vi "Main_ConfigDialog.vi"(8 "error in (no error)":errorcluster, 9 "boot path":path, 10 "Current project Path":path) -> (0 "error out":errorcluster)   [LabVIEW 2011]
uses:
  signal type.ctl
  gain.ctl
  filter.ctl
  Power_config.ctl
  contable.ctl
  CHS.ctl
  singlechtype.ctl
  <vilib>/Utility/miscctls.llb/LVPositionTypeDef.ctl
  config table enum.ctl
  config opr.ctl
panel:
  out "Numeric":i32
  out "size(s)":i32
  in  "LED":bool
  in  "threshold":dbl
  in  "CALclass":T1
  in  "PHName":string(combo)
  in  "ClassII":string
  in  "ClassI":string
  in  "boardName":string
  in  "Ch":u8
  in  "CNO":u8
  in  "Cluster":T2 {"CHS"."display" format="%b"}
  in  "Load":bool
  in  "Power":T5
  in  "Filter":T6={"en"=FALSE, "value"=10, "Boolean"=FALSE} caption="滤波"
  in  "Gain":T7
  in  "compare":T1
  in  "Apply":bool
  in  "sensorName":string(combo)
  in  "rate":dbl
  in  "alarm":string(combo)
  in  "enable":string(combo)
  in  "b":dbl
  in  "k":dbl
  in  "unit":string(combo)="A"
  in  "Etype":string(combo)="温度"
  in  "ChannalName":string
  in  "ChannalConfig":string(tree)
  in  "OK":bool
  in  "Save as":bool
  in  "Cancel":bool
  # "通道参数配置表"
  # "Ssdsa"
  # "Hz"
  # "Hz"
  # "Hz"
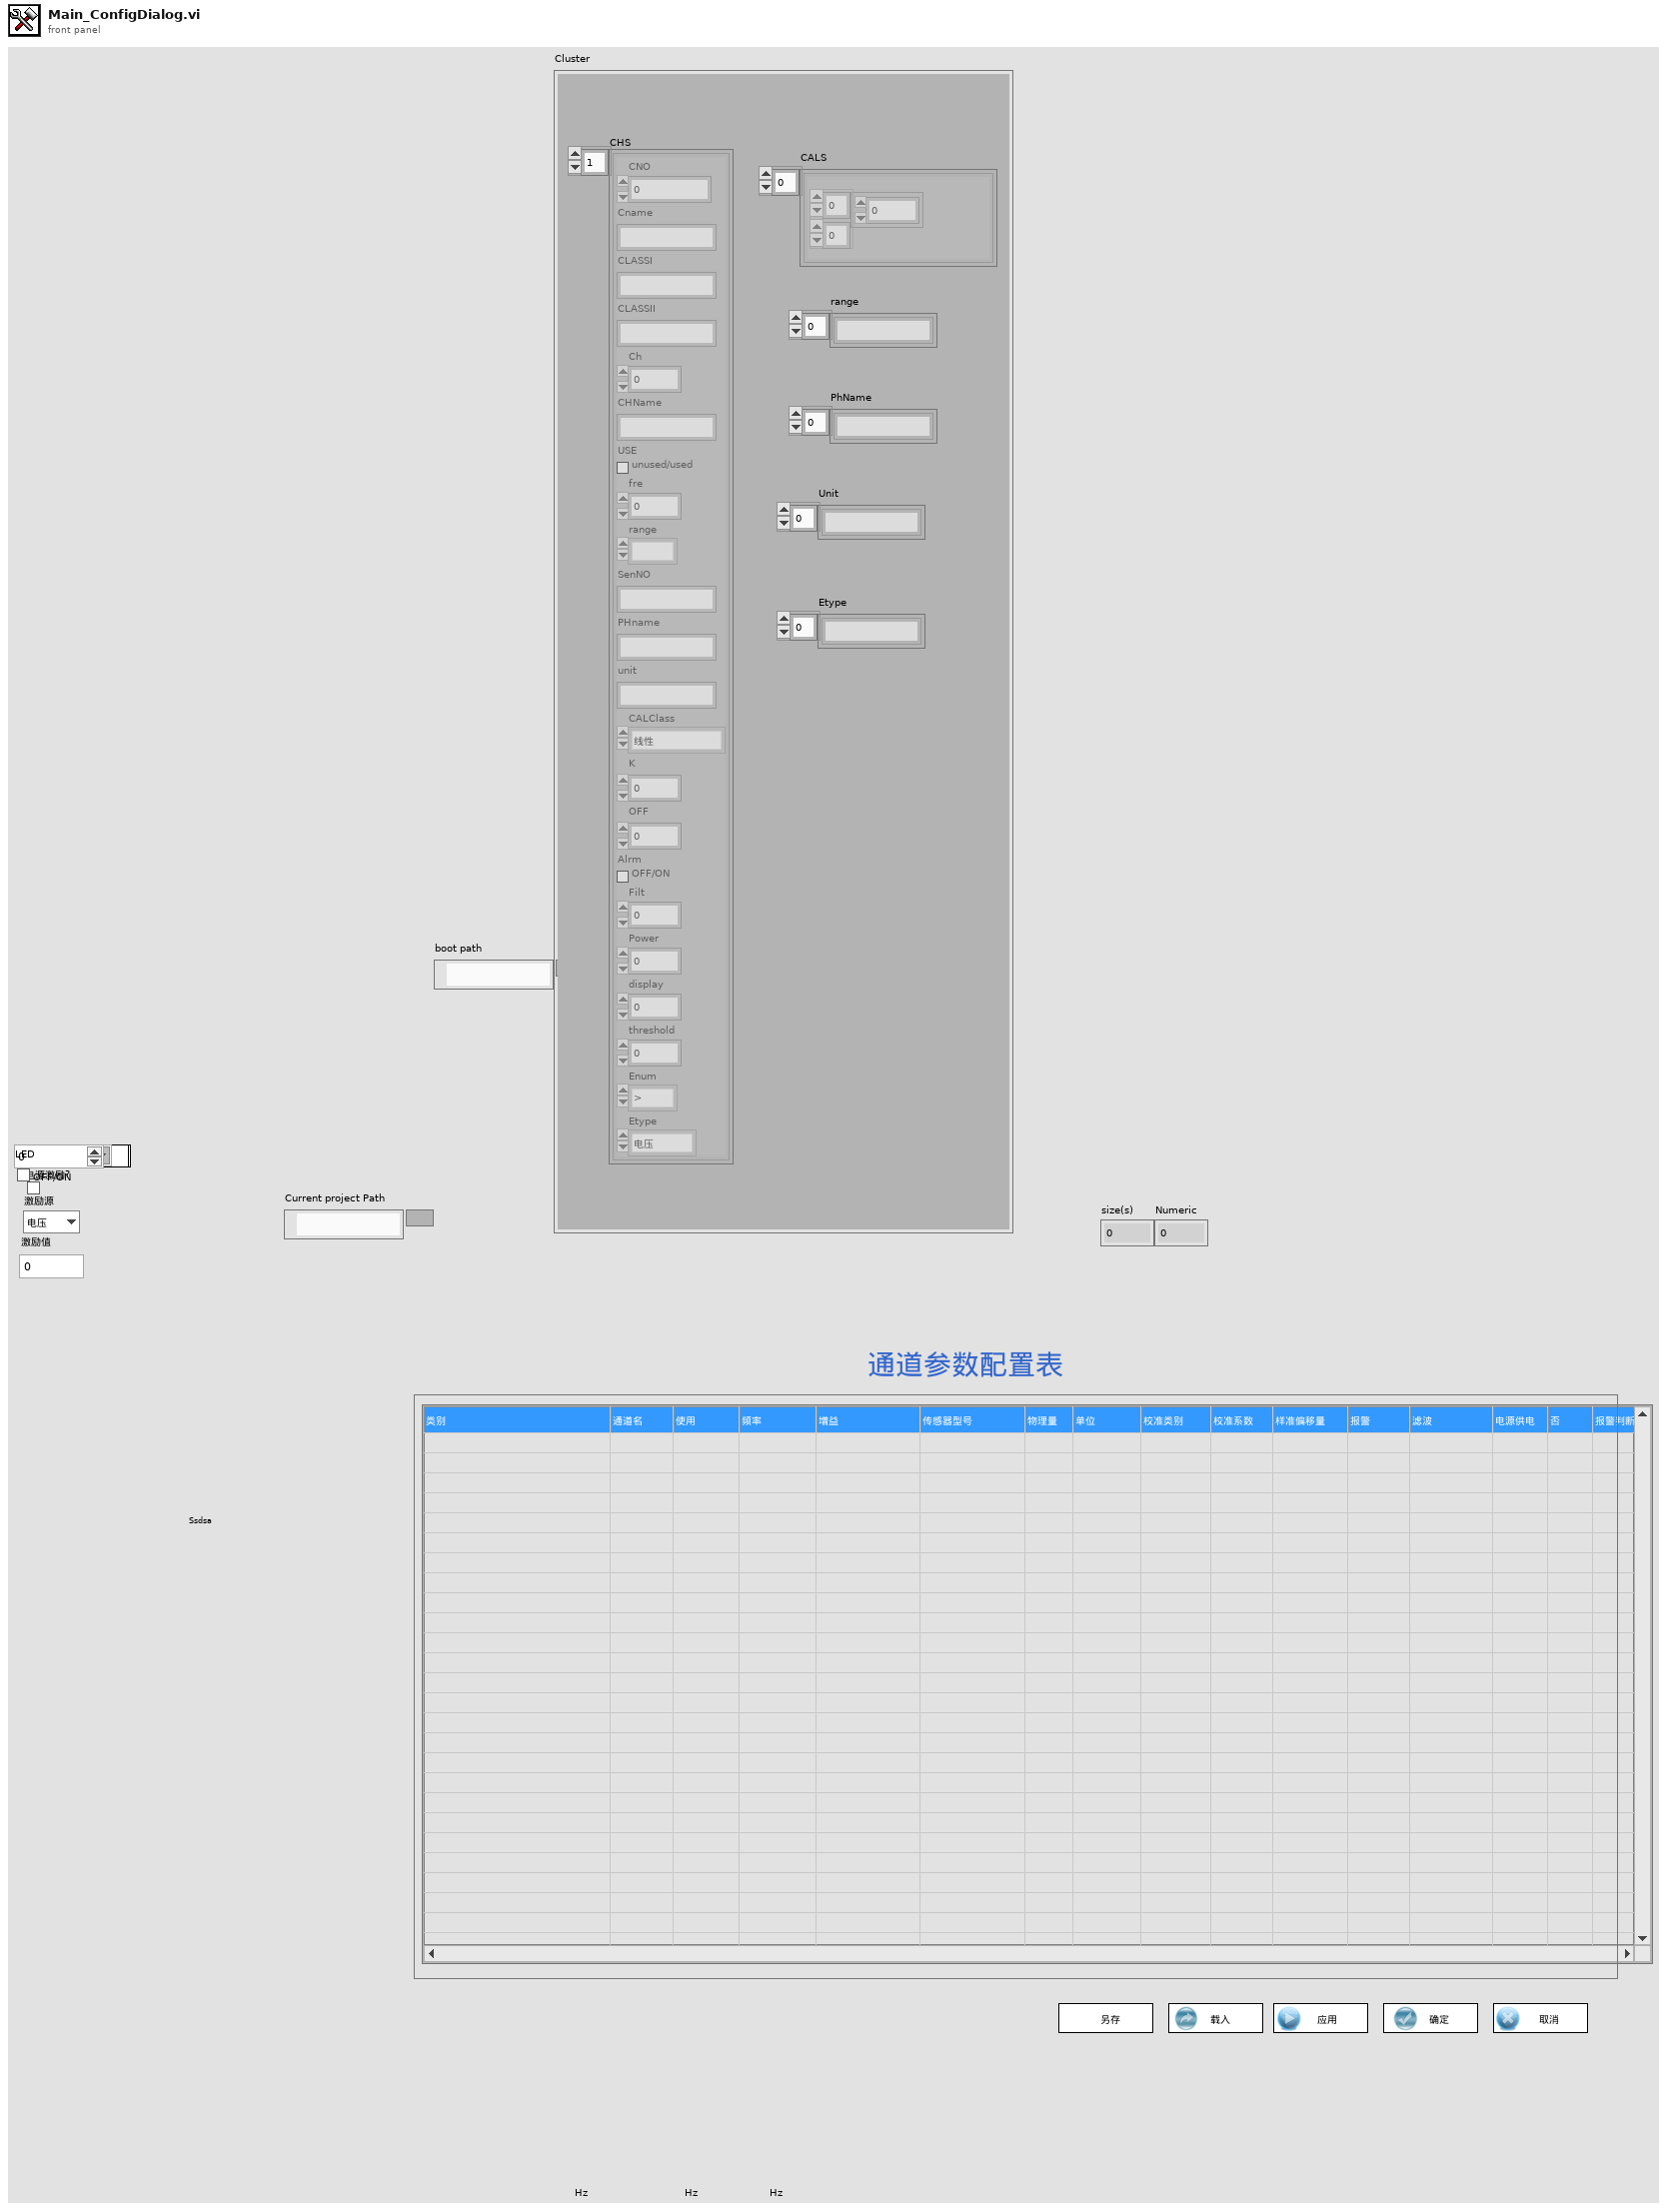
[diagram p1: front panel]
types:
  T1 = typedef "signal type.ctl" = enum16{"未设置", "volet", "current", "vibration", "electric charge ", "resistance "}
  T2 = typedef "contable.ctl" = cluster{"CHS":T3, "CALS":cluster{"Array":dbl[][]}[], "range":string[], "PhName":string[], "Unit":string[], "Etype":string[]}
  T3 = typedef "CHS.ctl" = T4[]
  T4 = typedef "singlechtype.ctl" = cluster{"CNO":u8, "Cname":string, "CLASSI":string, "CLASSII":string, "Ch":u8, "CHName":string, "USE":bool, "fre":dbl, "range":enum16{""}, "SenNO":string, "PHname":string, "unit":string, "CALClass":enum8{"线性", "查表", "公式"}, "K":dbl, "OFF":dbl, "Alrm":bool, "Filt":dbl, "Power":u8, "display":u8, "threshold ":dbl, "Enum":enum16{">", ">=", "<", "<=", "<>(在范围内）", "><（在范围外）"}, "Etype":enum16{"电压", "电流", "电阻", "热电偶K", "热电偶T"}}
  T5 = typedef "Power_config.ctl" = cluster{"power_en":bool, "Mode":enum16{"电压", "电流"}, "value":dbl, "Boolean":bool}
  T6 = typedef "filter.ctl" = cluster{"en":bool, "value":i32, "Boolean":bool}
  T7 = typedef "gain.ctl" = enum16{"±10V", "±5V", "±2.5V", "±1V", "±500mV", "±100mV", "10V", "5V", "2.5V", "1V", "500mV", "100mV"}
  T8 = typedef "LVPositionTypeDef.ctl" = cluster{"Left":i32, "Top":i32}
  T9 = typedef "config opr.ctl" = enum16{"new config", "read config", "write config", "close config", "write defaultconfig", ""}
  T10 = typedef "config table enum.ctl" = enum16{"CNO.", "CName", "CLASSI", "CLASSII", "ch", "Chname", "USE", "fre", "range", "senNO", "PHname", "unit", "CALclass", "K", "OFF", "Alrm", "filt", "Power", "display", "threshold", "compare", "Etype"}
  T11 = typedef "LVPoint32TypeDef.ctl" = cluster{"Horizontal":i32, "Vertical":i32}
  T12 = cluster{"manner":enum16{"线性", "查表"}, "data":dbl[][]}
  T13 = cluster{"manner":enum16{"线性", "查表"}, "data":dbl[][], "slop":dbl, "intercept":dbl, "sensorID":string, "signal type":string, "unit":string}
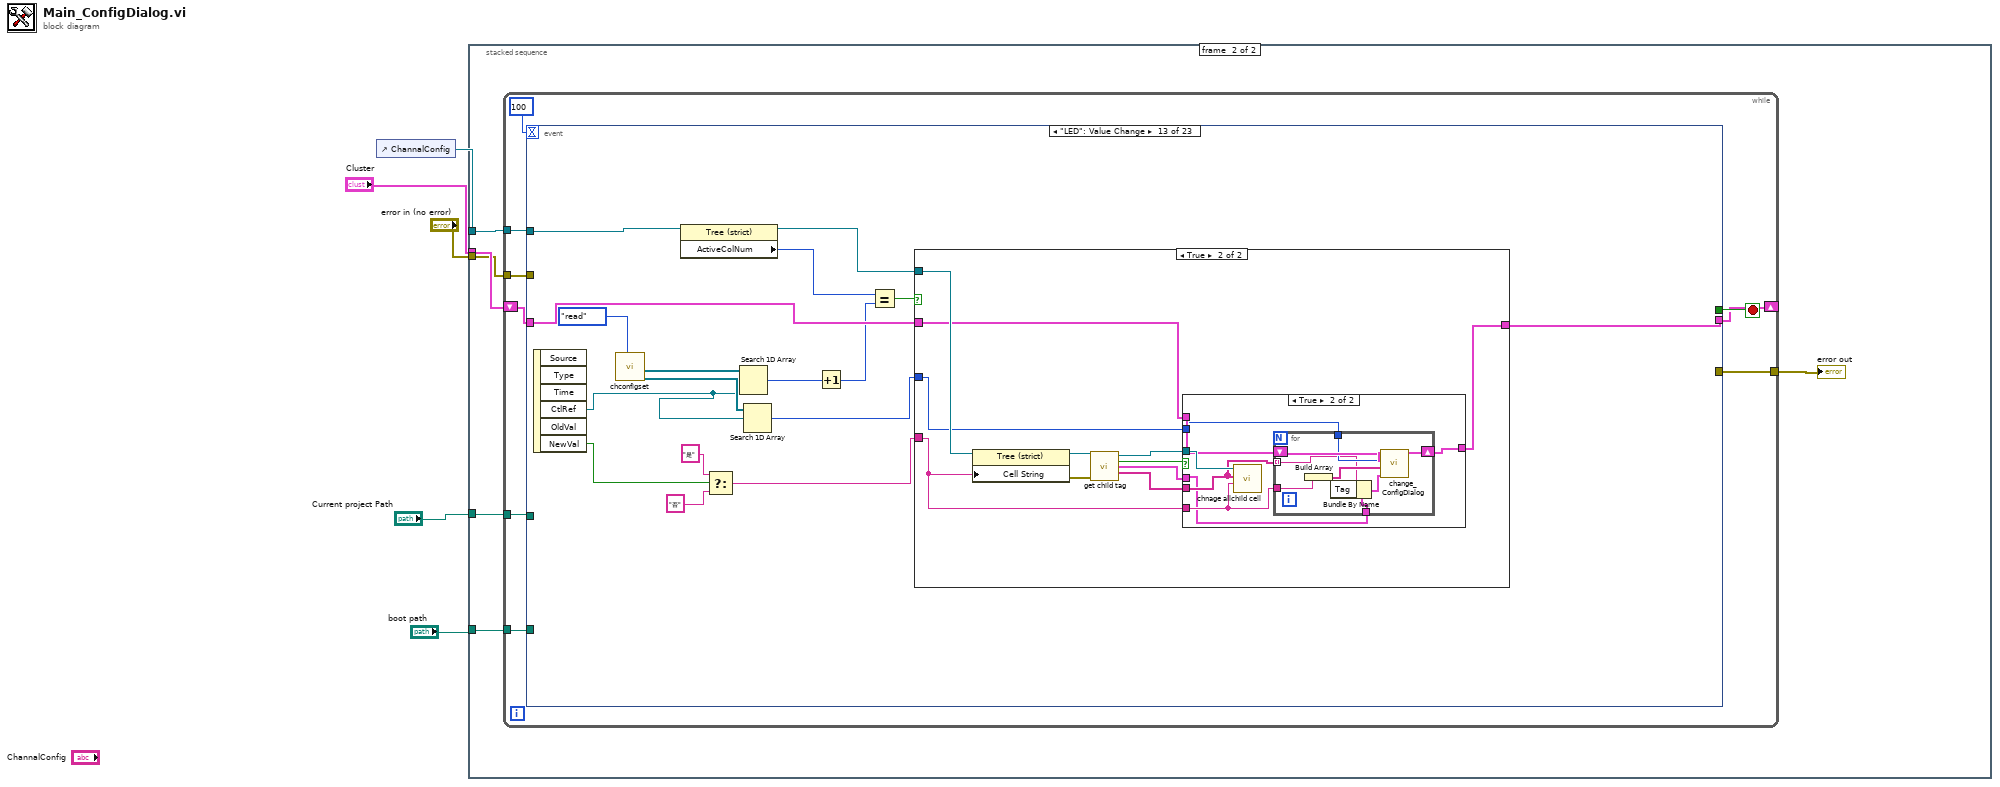
[diagram p0: block diagram]
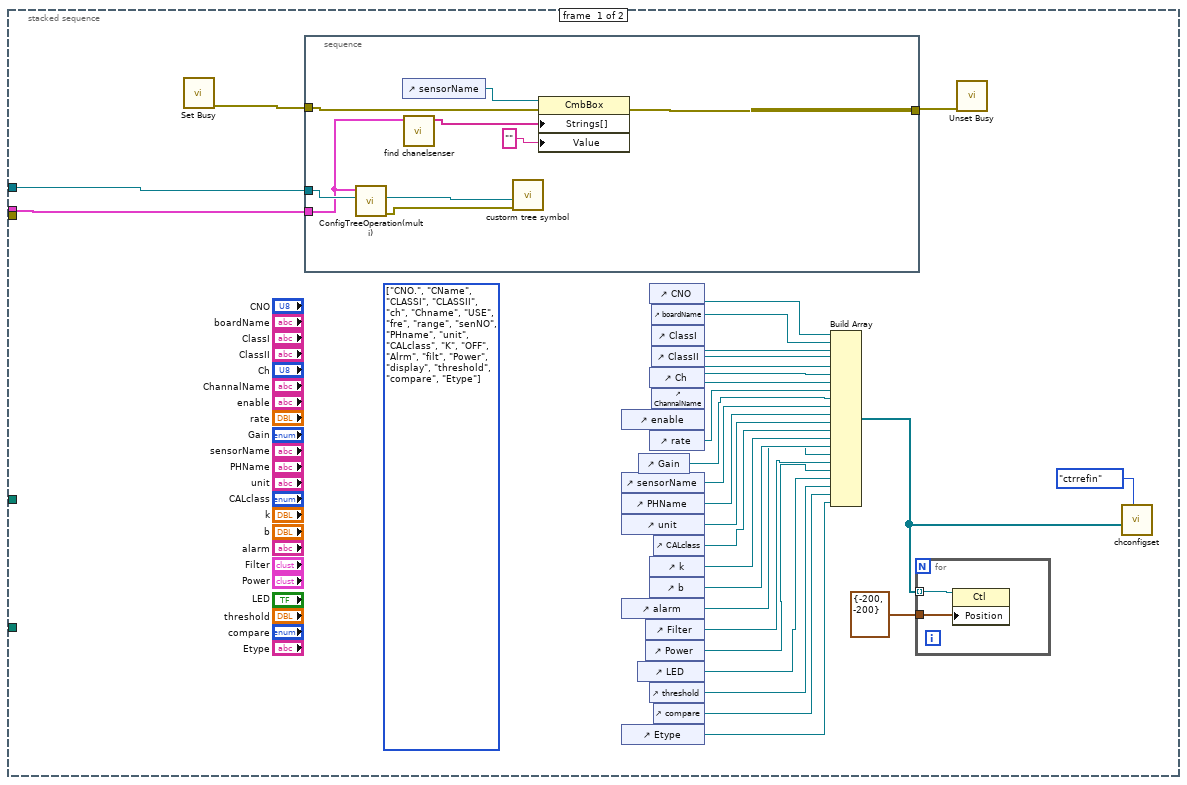
[diagram p2: hidden frame]
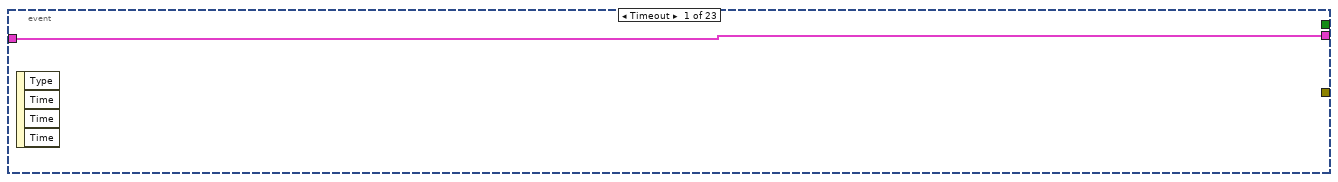
[diagram p3: hidden frame]
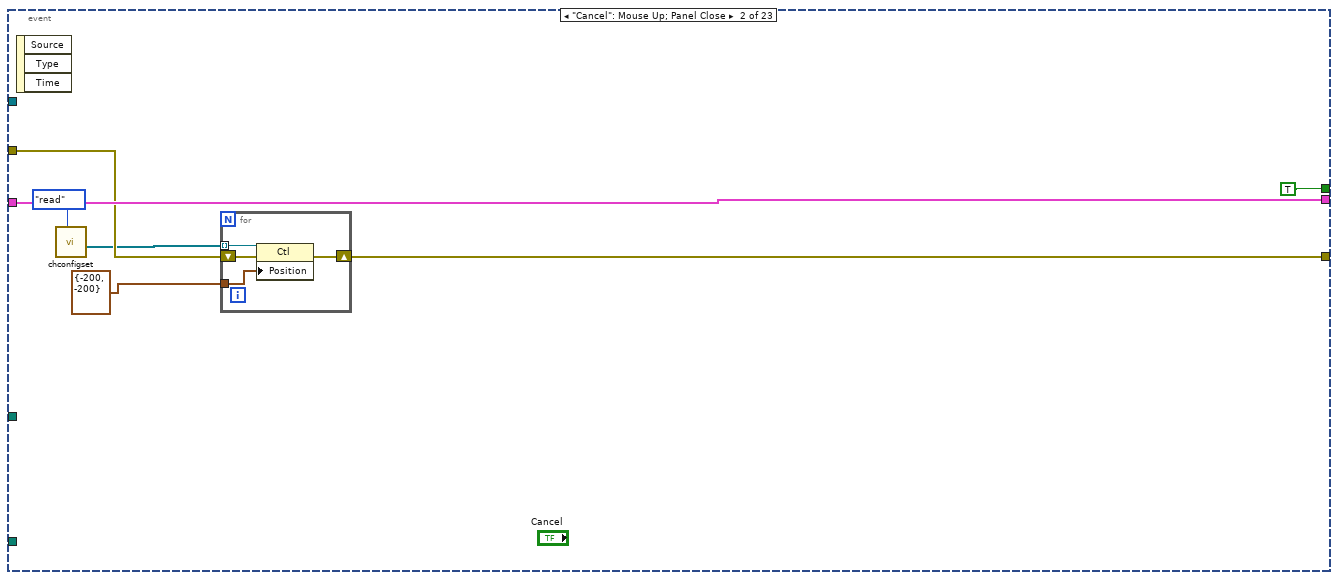
[diagram p4: hidden frame]
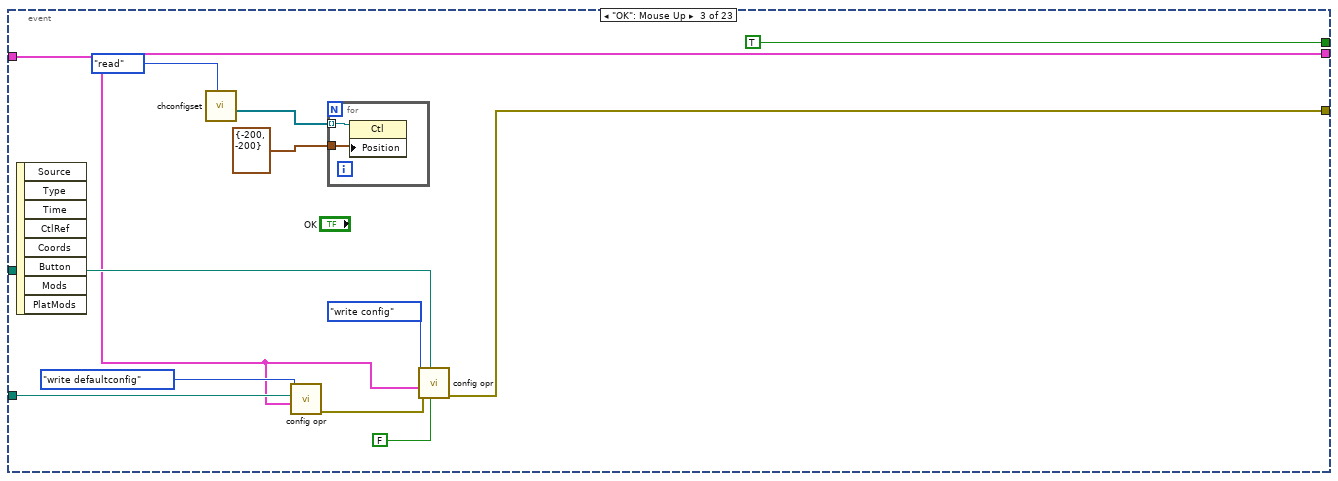
[diagram p5: hidden frame]
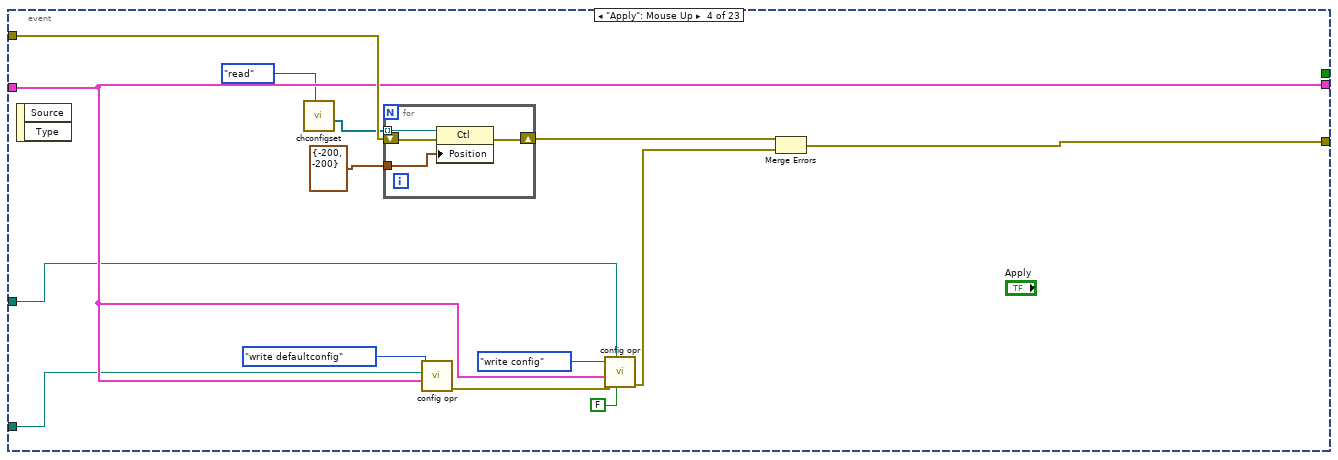
[diagram p6: hidden frame]
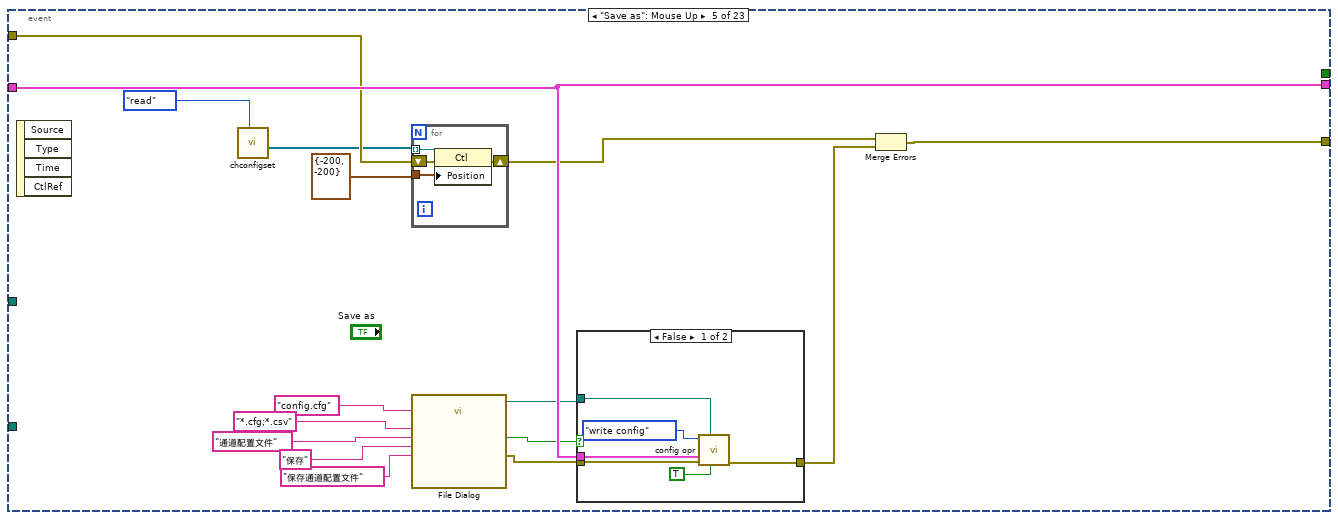
[diagram p7: hidden frame]
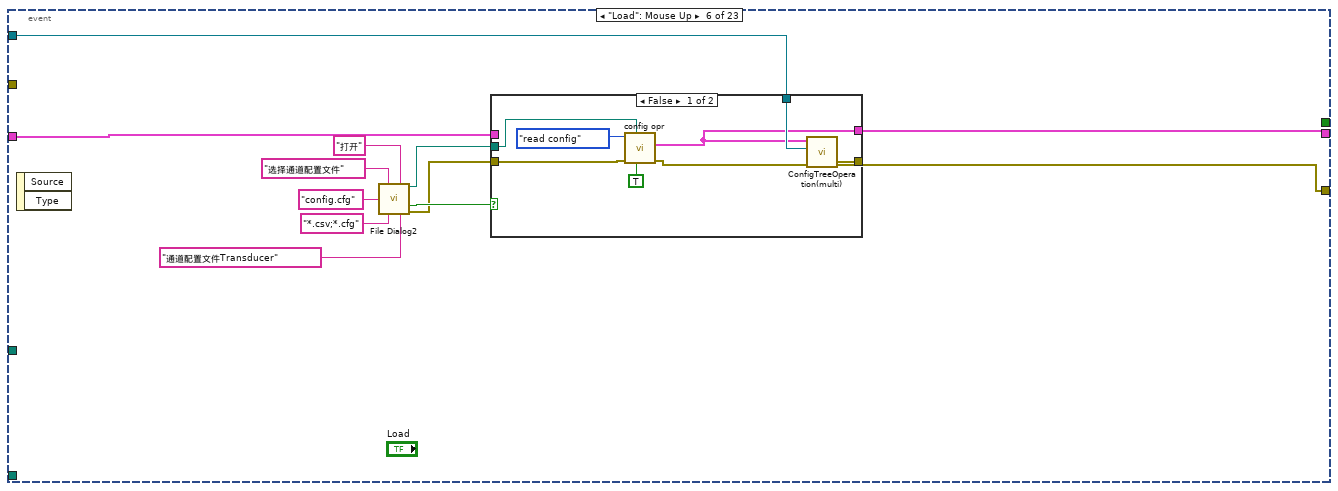
[diagram p9: hidden frame]
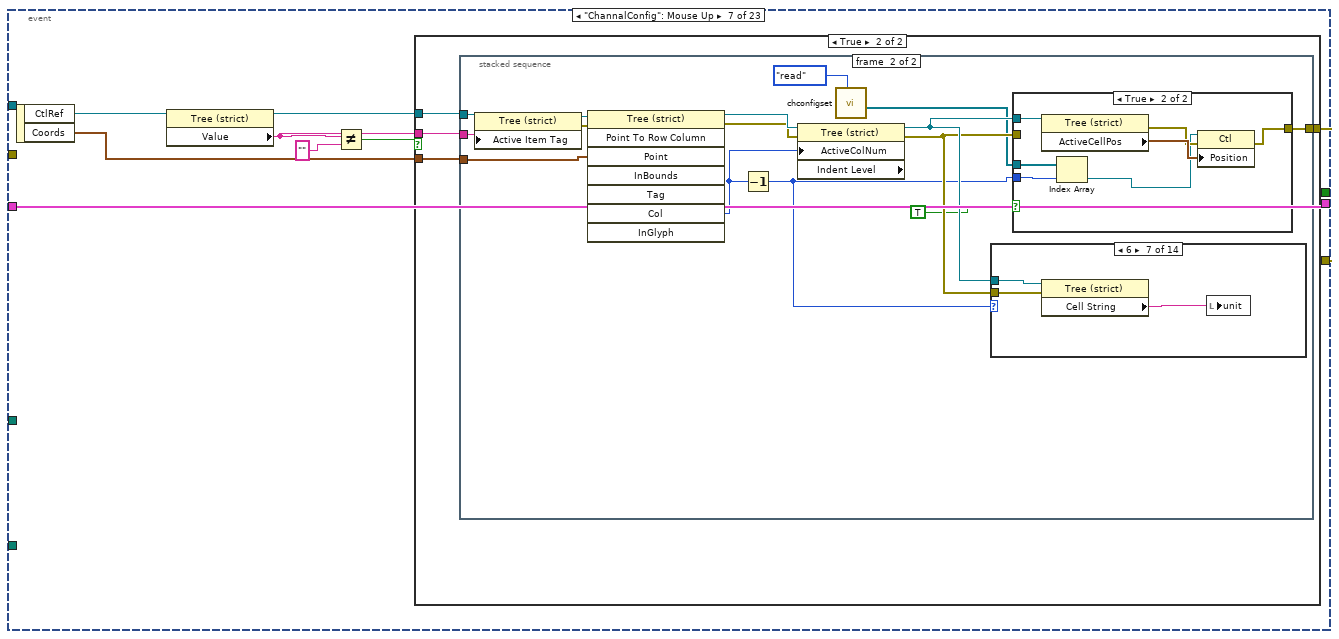
[diagram p11: hidden frame]
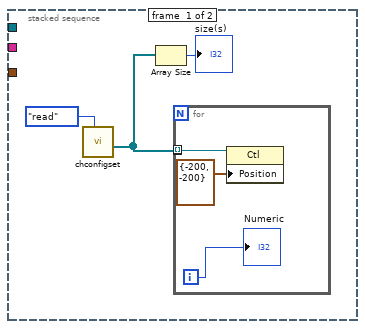
[diagram p13: hidden frame]
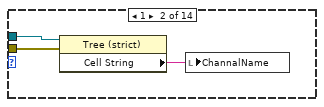
[diagram p16: hidden frame]
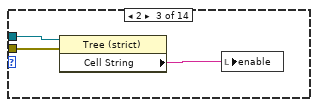
[diagram p17: hidden frame]
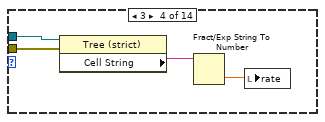
[diagram p18: hidden frame]
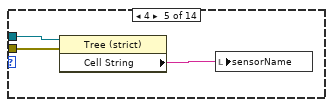
[diagram p19: hidden frame]
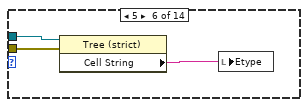
[diagram p20: hidden frame]
diagram:
  n1 = control-ref of="ChannalConfig"() -> (w5:refnum<vi>)
  n2 = stacked-sequence {
    tunnel: "Cluster" -> [w33 w51]
    tunnel: "error in (no error)" -> [_ w47]
    tunnel: w5 -> [w32 w50]
    tunnel: "Current project Path" -> [_ w49]
    tunnel: "boot path" -> [_ w46]
    frame #0 {
      (unwired) T10[] [enum."CNO.", enum."CName", enum."CLASSI", enum."CLASSII", enum."ch", enum."Chname", enum."USE", enum."fre", enum."range", enum."senNO", enum."PHname", enum."unit", enum."CALclass", enum."K", enum."OFF", enum."Alrm", enum."filt", enum."Power", enum."display", enum."threshold", enum."compare", enum."Etype"] items=["CNO.", "CName", "CLASSI", "CLASSII", "ch", "Chname", "USE", "fre", "range", "senNO", "PHname", "unit", "CALclass", "K", "OFF", "Alrm", "filt", "Power", "display", "threshold", "compare", "Etype"]
      n3 = call <vilib>:"Set Busy.vi"() -> ("error out"=w31:errorcluster)  [unwired: 4 in, 7 out]
      n4 = stacked-sequence {
        tunnel: w33 -> [w36]
        tunnel: w32 -> [w40]
        tunnel: w31 -> [w39]
        tunnel: [w38] -> w30
        frame #0 {
          n5 = call "ConfigTreeOperation(multi).vi"("Tree Refnum"=w40, "configtable"=w36) -> ("error out"=w35:errorcluster, "Tree Refnum out"=w37:refnum<vi>)  [unwired: 1 in, 7 out]
          n6 = control-ref of="sensorName"() -> (w41:refnum<vi>)
          n7 = call "find chanelsenser.vi"("configtable"=w36) -> ("senser out"=w43:string[])  [unwired: 10 out]
          n8 = call "custorm tree symbol.vi"("error in (no error)"=w35, "reference"=w37) -> ()  [unwired: 10 out]
          n9 = property class="CmbBox"(reference=w41, error in=w39, "Strings[]"=w43, "Value"="") -> (error out=w38:errorcluster)  [unwired: 1 out]
        }
      }
      n10 = control-ref of="enable"() -> (w21:refnum<vi>)
      n11 = control-ref of="sensorName"() -> (w10:refnum<vi>)
      n12 = control-ref of="PHName"() -> (w19:refnum<vi>)
      n13 = control-ref of="unit"() -> (w18:refnum<vi>)
      n14 = control-ref of="alarm"() -> (w13:refnum<vi>)
      n15 = control-ref of="Etype"() -> (w7:refnum<vi>)
      n16 = control-ref of="LED"() -> (w12:refnum<vi>)
      n17 = control-ref of="Gain"() -> (w6:refnum<vi>)
      n18 = control-ref of="Filter"() -> (w11:refnum<vi>)
      n19 = control-ref of="Power"() -> (w14:refnum<vi>)
      n20 = control-ref of="CNO"() -> (w27:refnum<vi>)
      n21 = control-ref of="Ch"() -> (w23:refnum<vi>)
      n22 = control-ref of="rate"() -> (w20:refnum<vi>)
      n23 = control-ref of="k"() -> (w16:refnum<vi>)
      n24 = control-ref of="b"() -> (w15:refnum<vi>)
      n25 = control-ref of="threshold"() -> (w9:refnum<vi>)
      n26 = control-ref of="boardName"() -> (w26:refnum<vi>)
      n27 = control-ref of="ClassI"() -> (w25:refnum<vi>)
      n28 = control-ref of="ClassII"() -> (w24:refnum<vi>)
      n29 = control-ref of="ChannalName"() -> (w22:refnum<vi>)
      n30 = control-ref of="CALclass"() -> (w17:refnum<vi>)
      n31 = control-ref of="compare"() -> (w8:refnum<vi>)
      n32 = Build Array(w27, w26, w25, w24, w23, w22, w21, w20, w6, w10, w19, w18, w17, w16, w15, w13, w11, w14, w12, w9, w8, w7) -> (w29:refnum<vi>[])
      n33 = for {
        tunnel: w29 -> [w45] mode=indexing
        tunnel: T8 {"Left"=-200, "Top"=-200} ("Position 3") -> [w44]
        n34 = property class="Ctl"(reference=w45, "Position"=w44) -> ()  [unwired: 1 in, 2 out]
      }
      n35 = call <vilib>:"Unset Busy.vi"("error in (no error)"=w30) -> ()  [unwired: 1 in, 10 out]
      n36 = call "chconfigset.vi"("Enum"=enum16{"init", "read", "treeheader", "ctrrefin"}."ctrrefin", "ref"=w29) -> ()  [unwired: 6 in, 4 out]
    }
    frame #1 {
      n37 = while {
        tunnel: w50 -> [w59]
        shift-right: [w56] -> _
        shift-left: w51 -> [w57]
        tunnel: w49 -> [w55]
        tunnel: [w54] -> w48
        tunnel: w47 -> [w53]
        tunnel: w46 -> [w52]
        stop <- w60 stop-if-true
        n38 = event shown="[12] \"LED\": Value Change" {
          selector: _ -> [_ _ _ _ _ _ _ _ _ _ _ _ _ _ _ _ _ _ _ _ _ _ _]
          dyn-events: _ -> [_ _ _ _ _ _ _ _ _ _ _ _ _ _ _ _ _ _ _ _ _ _ _]
          timeout: 100 -> [_ _ _ _ _ _ _ _ _ _ _ _ _ _ _ _ _ _ _ _ _ _ _]
          tunnel: [_ TRUE TRUE _ _ _ _ _ _ _ _ _ _ _ _ _ _ _ _ _ _ _ _] -> w60
          tunnel: w59 -> [_ _ _ _ _ w134 _ w248 w296 w343 w392 w439 w489 w538 w588 w644 w706 w774 w823 w872 w919 w965 _]
          tunnel: w57 -> [w61 w67 w75 w93 w114 w136 w155 w251 w298 w345 w394 w441 w491 w540 w590 w646 w708 w776 w825 w874 w921 w968 w1091]
          tunnel: [w61 w67 w75 w93 w114 w132 w155 w249 w297 w344 w393 w440 w490 w539 w589 w645 w707 w775 w824 w873 w920 w966 w1091] -> w56
          tunnel: w55 -> [_ _ w82 w92 _ _ _ _ _ _ _ _ _ _ _ _ _ _ _ _ _ w959 _]
          tunnel: [_ w64 w80 w90 w107 w133 w154 _ _ _ _ _ _ _ _ _ _ _ _ _ _ _ _] -> w54
          tunnel: w53 -> [_ w65 _ w99 w110 _ _ _ _ _ _ _ _ _ _ _ _ _ _ _ _ _ _]
          tunnel: w52 -> [_ _ w77 w91 _ _ _ _ _ _ _ _ _ _ _ _ _ _ _ _ _ w957 _]
          event Timeout {
            n39 = event-data() -> ()  [unwired: 5 out]
          }
          event "Cancel": Mouse Up; Panel Close {
            n40 = event-data() -> ()  [unwired: 4 out]
            n41 = call "chconfigset.vi"("Enum"=enum16{"init", "read", "treeheader", "ctrrefin"}."read") -> ("ref out"=w63:refnum<vi>[])  [unwired: 7 in, 3 out]
            n42 = for {
              tunnel: w63 -> [w72] mode=indexing
              tunnel: T8 {"Left"=-200, "Top"=-200} ("Position 3") -> [w71]
              shift-right: [w69] -> w64
              shift-left: w65 -> [w70]
              n43 = property class="Ctl"(reference=w72, error in=w70, "Position"=w71) -> (error out=w69:errorcluster)  [unwired: 1 out]
            }
          }
          event "OK": Mouse Up {
            n44 = event-data() -> ()  [unwired: 9 out]
            n45 = call "chconfigset.vi"("Enum"=enum16{"init", "read", "treeheader", "ctrrefin"}."read") -> ("ref out"=w74:refnum<vi>[])  [unwired: 7 in, 3 out]
            n46 = call "config opr.vi"("Chanel"=w75, "defaultPath"=w77, "config opr"=config_opr."write defaultconfig") -> ("error out"=w78:errorcluster)  [unwired: 5 in, 3 out]
            n47 = for {
              tunnel: w74 -> [w86] mode=indexing
              tunnel: T8 {"Left"=-200, "Top"=-200} ("Position 3") -> [w85]
              n48 = property class="Ctl"(reference=w86, "Position"=w85) -> ()  [unwired: 1 in, 2 out]
            }
            n49 = call "config opr.vi"("Not project Path?"=FALSE ("project Path?"), "project path"=w82, "error in"=w78, "Chanel"=w75, "config opr"=config_opr."write config") -> ("error out"=w80:errorcluster)  [unwired: 3 in, 3 out]
          }
          event "Apply": Mouse Up {
            n50 = event-data() -> ()  [unwired: 3 out]
            n51 = call "chconfigset.vi"("Enum"=enum16{"init", "read", "treeheader", "ctrrefin"}."read") -> ("ref out"=w88:refnum<vi>[])  [unwired: 7 in, 3 out]
            n52 = for {
              tunnel: T8 {"Left"=-200, "Top"=-200} ("Position 3") -> [w104]
              tunnel: w88 -> [w103] mode=indexing
              shift-right: [w101] -> w98
              shift-left: w99 -> [w102]
              n53 = property class="Ctl"(reference=w103, error in=w102, "Position"=w104) -> (error out=w101:errorcluster)  [unwired: 1 out]
            }
            n54 = call "config opr.vi"("Chanel"=w93, "defaultPath"=w91, "config opr"=config_opr."write defaultconfig") -> ("error out"=w95:errorcluster)  [unwired: 5 in, 3 out]
            n55 = call "config opr.vi"("Not project Path?"=FALSE ("project Path?"), "project path"=w92, "error in"=w95, "Chanel"=w93, "config opr"=config_opr."write config") -> ("error out"=w89:errorcluster)  [unwired: 3 in, 3 out]
            n56 = Merge Errors(w98, w89) -> (w90:errorcluster)
          }
          event "Save as": Mouse Up {
            n57 = event-data() -> ()  [unwired: 5 out]
            n58 = call "chconfigset.vi"("Enum"=enum16{"init", "read", "treeheader", "ctrrefin"}."read") -> ("ref out"=w106:refnum<vi>[])  [unwired: 7 in, 3 out]
            n59 = for {
              tunnel: w106 -> [w124] mode=indexing
              tunnel: T8 {"Left"=-200, "Top"=-200} ("Position 3") -> [w123]
              shift-right: [w121] -> w109
              shift-left: w110 -> [w122]
              n60 = property class="Ctl"(reference=w124, error in=w122, "Position"=w123) -> (error out=w121:errorcluster)  [unwired: 1 out]
            }
            n61 = call "File Dialog"("prompt"="保存通道配置文件", "button label"="保存", "default name"="config.cfg" ("pattern (all files)"), "pattern (all files)"="*.cfg;*.csv", "pattern label"="通道配置文件" ("default name")) -> ("selected path"=w112:path, "cancelled"=w113:bool, "error out"=w115:errorcluster)  [unwired: 2 in, 6 out]
            n62 = case shown="False" w113 {
              tunnel: w115 -> [w130 w131]
              tunnel: w114 -> [w129 _]
              tunnel: w112 -> [w128 _]
              tunnel: [w127 w131] -> w108
              frame False {
                n63 = call "config opr.vi"("Not project Path?"=TRUE, "project path"=w128, "error in"=w130, "Chanel"=w129, "config opr"=config_opr."write config") -> ("error out"=w127:errorcluster)  [unwired: 3 in, 3 out]
              }
              frame True {
              }
            }
            n64 = Merge Errors(w109, w108) -> (w107:errorcluster)
          }
          event "Load": Mouse Up {
            n65 = event-data() -> ()  [unwired: 3 out]
            n66 = call "File Dialog2"("prompt"="选择通道配置文件", "button label"="打开", "default name"="config.cfg" ("pattern (all files)"), "pattern (all files)"="*.csv;*.cfg", "pattern label"="通道配置文件Transducer" ("default name")) -> ("selected path"=w140:path, "cancelled"=w141:bool, "error out"=w135:errorcluster)  [unwired: 2 in, 6 out]
            n67 = case shown="False" w141 {
              tunnel: w140 -> [w149 _]
              tunnel: [w144 w153] -> w132
              tunnel: w136 -> [_ w153]
              tunnel: [w146 w152] -> w133
              tunnel: w135 -> [w150 w152]
              tunnel: w134 -> [w147 _]
              frame False {
                n68 = call "config opr.vi"("Not project Path?"=TRUE, "project path"=w149, "error in"=w150, "config opr"=config_opr."read config") -> ("error out"=w145:errorcluster, "chconfig data"=w144:T2)  [unwired: 4 in, 2 out]
                n69 = call "ConfigTreeOperation(multi).vi"("error in (no error)"=w145, "Tree Refnum"=w147, "configtable"=w144) -> ("error out"=w146:errorcluster)  [unwired: 8 out]
              }
              frame True {
              }
            }
          }
          event "ChannalConfig": Mouse Up {
            n70 = event-data() -> ("CtlRef"=w158:refnum<vi>, "Coords"=w161:T11)  [unwired: 1 out]
            n71 = property class="Tree (strict)"(reference=w158) -> (reference out=w156:refnum<vi>, "Value"=w157:string)  [unwired: 1 in, 1 out]
            n72 = Not Equal?(x=w157, y="") -> (x != y?=w159:bool)
            n73 = case shown="True" w159 {
              tunnel: w161 -> [_ w165]
              tunnel: w157 -> [_ w164]
              tunnel: w156 -> [_ w163]
              tunnel: [_ w162] -> w154
              frame False {
              }
              frame True {
                n74 = stacked-sequence {
                  tunnel: w165 -> [_ w183]
                  tunnel: w164 -> [_ w185]
                  tunnel: w163 -> [_ w180]
                  tunnel: [_ w177] -> w162
                  frame #0 {
                    n75 = call "chconfigset.vi"("Enum"=enum16{"init", "read", "treeheader", "ctrrefin"}."read") -> ("ref out"=w167:refnum<vi>[])  [unwired: 7 in, 3 out]
                    n76 = Array Size(array=w167) -> (size(s)=→"size(s)":i32)
                    n77 = for {
                      tunnel: w167 -> [w171] mode=indexing
                      tunnel: [w171] -> _ mode=indexing
                      i -> [w169]
                      n78 = property class="Ctl"(reference=w171, "Position"=T8 {"Left"=-200, "Top"=-200} ("Position 2")) -> ()  [unwired: 1 in, 2 out]
                      "Numeric" <- w169
                    }
                  }
                  frame #1 {
                    n79 = property class="Tree (strict)"(reference=w180, "Active Item Tag"=w185) -> (reference out=w186:refnum<vi>, error out=w182:errorcluster)  [unwired: 1 in]
                    n80 = invoke class="Tree (strict)" method="Point To Row Column"(reference=w186, error in=w182, "Point"=w183) -> (reference out=w184:refnum<vi>, error out=w181:errorcluster, "Col"=w173:i32)  [unwired: 5 in, 5 out]
                    n81 = Decrement(x=w173) -> (x-1=w172:i32)
                    n82 = property class="Tree (strict)" props=["ActiveColNum", "Indent Level"](reference=w184, error in=w181, "ActiveColNum"=w173) -> (reference out=w179:refnum<vi>, error out=w178:errorcluster)  [unwired: 1 out]
                    n83 = call "chconfigset.vi"("Enum"=enum16{"init", "read", "treeheader", "ctrrefin"}."read") -> ("ref out"=w176:refnum<vi>[])  [unwired: 7 in, 3 out]
                    n84 = case shown="6" w172 {
                      tunnel: w179 -> [_ w195 w199 w203 w205 w209 w212 w216 w220 w223 w227 w231 w234 w237]
                      tunnel: w178 -> [_ w194 w198 w202 w204 w208 w211 w215 w219 w222 _ _ _ _]
                      frame 0, Default {
                      }
                      frame 1 {
                        n85 = property class="Tree (strict)"(reference=w195, error in=w194) -> ("Cell String"=w196:string)  [unwired: 2 out]
                        n86 = local write "ChannalName"(w196) -> ()
                      }
                      frame 2 {
                        n87 = property class="Tree (strict)"(reference=w199, error in=w198) -> ("Cell String"=w197:string)  [unwired: 2 out]
                        n88 = local write "enable"(w197) -> ()
                      }
                      frame 3 {
                        n89 = property class="Tree (strict)"(reference=w203, error in=w202) -> ("Cell String"=w201:string)  [unwired: 2 out]
                        n90 = Fract/Exp String To Number(string=w201) -> (number=w200:dbl)  [unwired: 4 out]
                        n91 = local write "rate"(w200) -> ()
                      }
                      frame 4 {
                        n92 = property class="Tree (strict)"(reference=w205, error in=w204) -> ("Cell String"=w206:string)  [unwired: 2 out]
                        n93 = local write "sensorName"(w206) -> ()
                      }
                      frame 5 {
                        n94 = property class="Tree (strict)"(reference=w209, error in=w208) -> ("Cell String"=w207:string)  [unwired: 2 out]
                        n95 = local write "Etype"(w207) -> ()
                      }
                      frame 6 {
                        n96 = property class="Tree (strict)"(reference=w212, error in=w211) -> ("Cell String"=w210:string)  [unwired: 2 out]
                        n97 = local write "unit"(w210) -> ()
                      }
                      frame 7 {
                        n98 = property class="Tree (strict)"(reference=w216, error in=w215) -> ("Cell String"=w213:string)  [unwired: 2 out]
                        n99 = Fract/Exp String To Number(string=w213) -> (number=w214:dbl)  [unwired: 1 in, 3 out]
                        n100 = local write "k"(w214) -> ()
                      }
                      frame 8 {
                        n101 = property class="Tree (strict)"(reference=w220, error in=w219) -> ("Cell String"=w217:string)  [unwired: 2 out]
                        n102 = Fract/Exp String To Number(string=w217) -> (number=w218:dbl)  [unwired: 4 out]
                        n103 = local write "b"(w218) -> ()
                      }
                      frame 9 {
                        n104 = property class="Tree (strict)"(reference=w223, error in=w222) -> ("Cell String"=w221:string)  [unwired: 2 out]
                        n105 = local write "alarm"(w221) -> ()
                      }
                      frame 10 {
                        n106 = property class="Tree (strict)"(reference=w227) -> ("Cell String"=w225:string)  [unwired: 1 in, 2 out]
                        n107 = property on="compare" class="Enum (strict)"() -> ("Strings []"=w226:string[])  [unwired: 2 in, 2 out]
                        n108 = Search 1D Array(1D array=w226, element=w225) -> (index of element=w224:i32)  [unwired: 1 out]
                        n109 = local write "compare"(w224) -> ()
                      }
                      frame 11 {
                        n110 = property class="Tree (strict)"(reference=w231) -> ("Cell String"=w229:string)  [unwired: 1 in, 2 out]
                        n111 = property on="Gain" class="Enum (strict)"() -> ("Strings []"=w230:string[])  [unwired: 2 in, 2 out]
                        n112 = Search 1D Array(1D array=w230, element=w229) -> (index of element=w228:i32)  [unwired: 1 out]
                        n113 = local write "Gain"(w228) -> ()
                      }
                      frame 12 {
                        n114 = property class="Tree (strict)"(reference=w234) -> ("Cell String"=w233:string)  [unwired: 1 in, 2 out]
                        n115 = call "string to power value.vi"("String"=w233) -> ("Power"=w232:T5)  [unwired: 14 out]
                        n116 = local write "Power"(w232) -> ()
                      }
                      frame 13 {
                        n117 = property class="Tree (strict)"(reference=w237) -> ("Cell String"=w236:string)  [unwired: 1 in, 2 out]
                        n118 = call "string to filter value.vi"("String"=w236) -> ("Filter Value"=w235:T6)  [unwired: 14 out]
                        n119 = local write "Filter"(w235) -> ()
                      }
                    }
                    n120 = case shown="True" TRUE {
                      tunnel: w176 -> [_ w193]
                      tunnel: w179 -> [_ w189]
                      tunnel: w172 -> [_ w191]
                      tunnel: w178 -> [_ _]
                      tunnel: [_ w188] -> w177
                      frame False {
                      }
                      frame True {
                        n121 = property class="Tree (strict)"(reference=w189) -> (error out=w190:errorcluster, "ActiveCellPos"=w192:T8)  [unwired: 1 in, 1 out]
                        n122 = Index Array(array=w193, index=w191) -> (element=w187:refnum<vi>)
                        n123 = property class="Ctl"(reference=w187, error in=w190, "Position"=w192) -> (error out=w188:errorcluster)  [unwired: 1 out]
                      }
                    }
                  }
                }
              }
            }
          }
          event "ChannalName": Value Change {
            n124 = event-data() -> ("CtlRef"=w241:refnum<vi>, "NewVal"=w250:string)  [unwired: 4 out]
            n125 = call "chconfigset.vi"("Enum"=enum16{"init", "read", "treeheader", "ctrrefin"}."read") -> ("All ref"=w242:refnum<vi>[], "ref out"=w244:refnum<vi>[])  [unwired: 7 in, 2 out]
            n126 = property class="Tree (strict)"(reference=w248) -> (reference out=w247:refnum<vi>, "ActiveColNum"=w246:i32)  [unwired: 1 in, 1 out]
            n127 = Search 1D Array(1D array=w244, element=w241) -> (index of element=w239:i32)  [unwired: 1 in]
            n128 = Search 1D Array(1D array=w242, element=w241) -> (index of element=w240:i32)  [unwired: 1 in]
            n129 = Increment(x=w239) -> (x+1=w238:i32)
            n130 = Equal?(x=w246, y=w238) -> (x = y?=w245:bool)
            n131 = case shown="True" w245 {
              tunnel: w251 -> [w252 w255]
              tunnel: w250 -> [_ w263]
              tunnel: [w252 w254] -> w249
              tunnel: w247 -> [_ w262]
              tunnel: w240 -> [_ w253]
              frame False {
              }
              frame True {
                n132 = property class="Tree (strict)"(reference=w262, "Cell String"=w263) -> (reference out=w260:refnum<vi>, error out=w261:errorcluster)  [unwired: 1 in]
                n133 = call "get child tag.vi"("ChannalConfig"=w260, "error in (no error)"=w261) -> ("ChannalConfig out"=w257:refnum<vi>, "? parent"=w259:bool, "tag and parent tag"=w256:cluster{"Tag":string, "Parent tag":string}, "child tag"=w258:string[])  [unwired: 10 out]
                n134 = case shown="True" w259 {
                  tunnel: w257 -> [_ w276]
                  tunnel: w258 -> [_ w275]
                  tunnel: w263 -> [w269 w271]
                  tunnel: w256 -> [w267 w270]
                  tunnel: w255 -> [w266 w273]
                  tunnel: [w265 w274] -> w254
                  tunnel: w253 -> [w264 w272]
                  frame False {
                    n135 = Build Array(w269) -> (w268:string[])
                    n136 = call "change_ConfigDialog.vi"("tag and parent tag"=w267, "value"=w268, "Enum"=w264, "configtable"=w266) -> ("all device out"=w265:T2)  [unwired: 1 in, 6 out]
                  }
                  frame True {
                    n137 = call "chnage allchild cell.vi"("Active Cell:String"=w271, "all childtag"=w275, "ChannalConfig"=w276) -> ()  [unwired: 9 out]
                    n138 = for {
                      tunnel: w275 -> [w277] mode=indexing
                      shift-right: [w284] -> w274
                      shift-left: w273 -> [w283]
                      tunnel: w272 -> [w282]
                      tunnel: w271 -> [w281]
                      tunnel: w270 -> [w279]
                      n139 = Build Array(w281) -> (w280:string[])
                      n140 = Bundle By Name(cluster=w279, "Tag"=w277) -> (w278:cluster{"Tag":string, "Parent tag":string})
                      n141 = call "change_ConfigDialog.vi"("tag and parent tag"=w278, "value"=w280, "Enum"=w282, "configtable"=w283) -> ("all device out"=w284:T2)  [unwired: 1 in, 6 out]
                    }
                  }
                }
              }
            }
          }
          event "PHName": Value Change {
            n142 = event-data() -> ("CtlRef"=w287:refnum<vi>, "NewVal"=w285:string)  [unwired: 5 out]
            n143 = call "chconfigset.vi"("Enum"=enum16{"init", "read", "treeheader", "ctrrefin"}."read") -> ("All ref"=w288:refnum<vi>[], "ref out"=w290:refnum<vi>[])  [unwired: 7 in, 2 out]
            n144 = property class="Tree (strict)"(reference=w296) -> (reference out=w295:refnum<vi>, "ActiveColNum"=w294:i32)  [unwired: 1 in, 1 out]
            n145 = Search 1D Array(1D array=w290, element=w287) -> (index of element=w293:i32)  [unwired: 1 in]
            n146 = Search 1D Array(1D array=w288, element=w287) -> (index of element=w286:i32)  [unwired: 1 in]
            n147 = Increment(x=w293) -> (x+1=w291:i32)
            n148 = Equal?(x=w294, y=w291) -> (x = y?=w292:bool)
            n149 = case shown="True" w292 {
              tunnel: w298 -> [w299 w302]
              tunnel: w285 -> [_ w310]
              tunnel: [w299 w301] -> w297
              tunnel: w295 -> [_ w309]
              tunnel: w286 -> [_ w300]
              frame False {
              }
              frame True {
                n150 = property class="Tree (strict)"(reference=w309, "Cell String"=w310) -> (reference out=w307:refnum<vi>, error out=w308:errorcluster)  [unwired: 1 in]
                n151 = call "get child tag.vi"("ChannalConfig"=w307, "error in (no error)"=w308) -> ("ChannalConfig out"=w304:refnum<vi>, "? parent"=w306:bool, "tag and parent tag"=w303:cluster{"Tag":string, "Parent tag":string}, "child tag"=w305:string[])  [unwired: 10 out]
                n152 = case shown="True" w306 {
                  tunnel: w304 -> [_ w323]
                  tunnel: w305 -> [_ w322]
                  tunnel: w310 -> [w316 w318]
                  tunnel: w303 -> [w314 w317]
                  tunnel: w302 -> [w313 w320]
                  tunnel: [w312 w321] -> w301
                  tunnel: w300 -> [w311 w319]
                  frame False {
                    n153 = Build Array(w316) -> (w315:string[])
                    n154 = call "change_ConfigDialog.vi"("tag and parent tag"=w314, "value"=w315, "Enum"=w311, "configtable"=w313) -> ("all device out"=w312:T2)  [unwired: 1 in, 6 out]
                  }
                  frame True {
                    n155 = call "chnage allchild cell.vi"("Active Cell:String"=w318, "all childtag"=w322, "ChannalConfig"=w323) -> ()  [unwired: 9 out]
                    n156 = for {
                      tunnel: w322 -> [w324] mode=indexing
                      shift-right: [w331] -> w321
                      shift-left: w320 -> [w330]
                      tunnel: w319 -> [w329]
                      tunnel: w318 -> [w328]
                      tunnel: w317 -> [w326]
                      n157 = Build Array(w328) -> (w327:string[])
                      n158 = Bundle By Name(cluster=w326, "Tag"=w324) -> (w325:cluster{"Tag":string, "Parent tag":string})
                      n159 = call "change_ConfigDialog.vi"("tag and parent tag"=w325, "value"=w327, "Enum"=w329, "configtable"=w330) -> ("all device out"=w331:T2)  [unwired: 1 in, 6 out]
                    }
                  }
                }
              }
            }
          }
          event "unit": Value Change {
            n160 = event-data() -> ("CtlRef"=w334:refnum<vi>, "NewVal"=w332:string)  [unwired: 5 out]
            n161 = call "chconfigset.vi"("Enum"=enum16{"init", "read", "treeheader", "ctrrefin"}."read") -> ("All ref"=w335:refnum<vi>[], "ref out"=w337:refnum<vi>[])  [unwired: 7 in, 2 out]
            n162 = property class="Tree (strict)"(reference=w343) -> (reference out=w342:refnum<vi>, "ActiveColNum"=w341:i32)  [unwired: 1 in, 1 out]
            n163 = Search 1D Array(1D array=w337, element=w334) -> (index of element=w340:i32)  [unwired: 1 in]
            n164 = Search 1D Array(1D array=w335, element=w334) -> (index of element=w333:i32)  [unwired: 1 in]
            n165 = Increment(x=w340) -> (x+1=w338:i32)
            n166 = Equal?(x=w341, y=w338) -> (x = y?=w339:bool)
            n167 = case shown="True" w339 {
              tunnel: w345 -> [w346 w349]
              tunnel: w332 -> [_ w357]
              tunnel: [w346 w348] -> w344
              tunnel: w342 -> [_ w356]
              tunnel: w333 -> [_ w347]
              frame False {
              }
              frame True {
                n168 = property class="Tree (strict)"(reference=w356, "Cell String"=w357) -> (reference out=w354:refnum<vi>, error out=w355:errorcluster)  [unwired: 1 in]
                n169 = call "get child tag.vi"("ChannalConfig"=w354, "error in (no error)"=w355) -> ("ChannalConfig out"=w351:refnum<vi>, "? parent"=w353:bool, "tag and parent tag"=w350:cluster{"Tag":string, "Parent tag":string}, "child tag"=w352:string[])  [unwired: 10 out]
                n170 = case shown="True" w353 {
                  tunnel: w351 -> [_ w370]
                  tunnel: w352 -> [_ w369]
                  tunnel: w357 -> [w363 w365]
                  tunnel: w350 -> [w361 w364]
                  tunnel: w349 -> [w360 w367]
                  tunnel: [w359 w368] -> w348
                  tunnel: w347 -> [w358 w366]
                  frame False {
                    n171 = Build Array(w363) -> (w362:string[])
                    n172 = call "change_ConfigDialog.vi"("tag and parent tag"=w361, "value"=w362, "Enum"=w358, "configtable"=w360) -> ("all device out"=w359:T2)  [unwired: 1 in, 6 out]
                  }
                  frame True {
                    n173 = call "chnage allchild cell.vi"("Active Cell:String"=w365, "all childtag"=w369, "ChannalConfig"=w370) -> ()  [unwired: 9 out]
                    n174 = for {
                      tunnel: w369 -> [w371] mode=indexing
                      shift-right: [w378] -> w368
                      shift-left: w367 -> [w377]
                      tunnel: w366 -> [w376]
                      tunnel: w365 -> [w375]
                      tunnel: w364 -> [w373]
                      n175 = Build Array(w375) -> (w374:string[])
                      n176 = Bundle By Name(cluster=w373, "Tag"=w371) -> (w372:cluster{"Tag":string, "Parent tag":string})
                      n177 = call "change_ConfigDialog.vi"("tag and parent tag"=w372, "value"=w374, "Enum"=w376, "configtable"=w377) -> ("all device out"=w378:T2)  [unwired: 1 in, 6 out]
                    }
                  }
                }
              }
            }
          }
          event Value Change {
            n178 = event-data() -> ("CtlRef"=w382:refnum<vi>, "NewVal"=w380:T1)  [unwired: 5 out]
            n179 = call "chconfigset.vi"("Enum"=enum16{"init", "read", "treeheader", "ctrrefin"}."read") -> ("All ref"=w384:refnum<vi>[], "ref out"=w386:refnum<vi>[])  [unwired: 7 in, 2 out]
            n180 = property class="Enum (strict)"(reference=w382) -> ("Strings []"=w381:string[])  [unwired: 1 in, 2 out]
            n181 = property class="Tree (strict)"(reference=w392) -> (reference out=w391:refnum<vi>, "ActiveColNum"=w390:i32)  [unwired: 1 in, 1 out]
            n182 = Search 1D Array(1D array=w386, element=w382) -> (index of element=w389:i32)  [unwired: 1 in]
            n183 = Search 1D Array(1D array=w384, element=w382) -> (index of element=w383:i32)  [unwired: 1 in]
            n184 = Index Array(array=w381, index=w380) -> (element=w379:string)
            n185 = Increment(x=w389) -> (x+1=w387:i32)
            n186 = Equal?(x=w390, y=w387) -> (x = y?=w388:bool)
            n187 = case shown="True" w388 {
              tunnel: w394 -> [w395 w398]
              tunnel: w379 -> [_ w406]
              tunnel: [w395 w397] -> w393
              tunnel: w391 -> [_ w405]
              tunnel: w383 -> [_ w396]
              frame False {
              }
              frame True {
                n188 = property class="Tree (strict)"(reference=w405, "Cell String"=w406) -> (reference out=w403:refnum<vi>, error out=w404:errorcluster)  [unwired: 1 in]
                n189 = call "get child tag.vi"("ChannalConfig"=w403, "error in (no error)"=w404) -> ("ChannalConfig out"=w400:refnum<vi>, "? parent"=w402:bool, "tag and parent tag"=w399:cluster{"Tag":string, "Parent tag":string}, "child tag"=w401:string[])  [unwired: 10 out]
                n190 = case shown="True" w402 {
                  tunnel: w400 -> [_ w419]
                  tunnel: w401 -> [_ w418]
                  tunnel: w406 -> [w412 w414]
                  tunnel: w399 -> [w410 w413]
                  tunnel: w398 -> [w409 w416]
                  tunnel: [w408 w417] -> w397
                  tunnel: w396 -> [w407 w415]
                  frame False {
                    n191 = Build Array(w412) -> (w411:string[])
                    n192 = call "change_ConfigDialog.vi"("tag and parent tag"=w410, "value"=w411, "Enum"=w407, "configtable"=w409) -> ("all device out"=w408:T2)  [unwired: 1 in, 6 out]
                  }
                  frame True {
                    n193 = call "chnage allchild cell.vi"("Active Cell:String"=w414, "all childtag"=w418, "ChannalConfig"=w419) -> ()  [unwired: 9 out]
                    n194 = for {
                      tunnel: w418 -> [w420] mode=indexing
                      shift-right: [w427] -> w417
                      shift-left: w416 -> [w426]
                      tunnel: w415 -> [w425]
                      tunnel: w414 -> [w424]
                      tunnel: w413 -> [w422]
                      n195 = Build Array(w424) -> (w423:string[])
                      n196 = Bundle By Name(cluster=w422, "Tag"=w420) -> (w421:cluster{"Tag":string, "Parent tag":string})
                      n197 = call "change_ConfigDialog.vi"("tag and parent tag"=w421, "value"=w423, "Enum"=w425, "configtable"=w426) -> ("all device out"=w427:T2)  [unwired: 1 in, 6 out]
                    }
                  }
                }
              }
            }
          }
          event "enable", "alarm": Value Change {
            n198 = event-data() -> ("CtlRef"=w430:refnum<vi>, "NewVal"=w428:string)  [unwired: 5 out]
            n199 = call "chconfigset.vi"("Enum"=enum16{"init", "read", "treeheader", "ctrrefin"}."read") -> ("All ref"=w431:refnum<vi>[], "ref out"=w433:refnum<vi>[])  [unwired: 7 in, 2 out]
            n200 = property class="Tree (strict)"(reference=w439) -> (reference out=w438:refnum<vi>, "ActiveColNum"=w437:i32)  [unwired: 1 in, 1 out]
            n201 = Search 1D Array(1D array=w433, element=w430) -> (index of element=w436:i32)  [unwired: 1 in]
            n202 = Search 1D Array(1D array=w431, element=w430) -> (index of element=w429:i32)  [unwired: 1 in]
            n203 = Increment(x=w436) -> (x+1=w434:i32)
            n204 = Equal?(x=w437, y=w434) -> (x = y?=w435:bool)
            n205 = case shown="True" w435 {
              tunnel: w441 -> [w442 w445]
              tunnel: w428 -> [_ w453]
              tunnel: [w442 w444] -> w440
              tunnel: w438 -> [_ w452]
              tunnel: w429 -> [_ w443]
              frame False {
              }
              frame True {
                n206 = property class="Tree (strict)"(reference=w452, "Cell String"=w453) -> (reference out=w450:refnum<vi>, error out=w451:errorcluster)  [unwired: 1 in]
                n207 = call "get child tag.vi"("ChannalConfig"=w450, "error in (no error)"=w451) -> ("ChannalConfig out"=w447:refnum<vi>, "? parent"=w449:bool, "tag and parent tag"=w446:cluster{"Tag":string, "Parent tag":string}, "child tag"=w448:string[])  [unwired: 10 out]
                n208 = case shown="True" w449 {
                  tunnel: w447 -> [_ w466]
                  tunnel: w448 -> [_ w465]
                  tunnel: w453 -> [w459 w461]
                  tunnel: w446 -> [w457 w460]
                  tunnel: w445 -> [w456 w463]
                  tunnel: [w455 w464] -> w444
                  tunnel: w443 -> [w454 w462]
                  frame False {
                    n209 = Build Array(w459) -> (w458:string[])
                    n210 = call "change_ConfigDialog.vi"("tag and parent tag"=w457, "value"=w458, "Enum"=w454, "configtable"=w456) -> ("all device out"=w455:T2)  [unwired: 1 in, 6 out]
                  }
                  frame True {
                    n211 = call "chnage allchild cell.vi"("Active Cell:String"=w461, "all childtag"=w465, "ChannalConfig"=w466) -> ()  [unwired: 9 out]
                    n212 = for {
                      tunnel: w465 -> [w467] mode=indexing
                      shift-right: [w474] -> w464
                      shift-left: w463 -> [w473]
                      tunnel: w462 -> [w472]
                      tunnel: w461 -> [w471]
                      tunnel: w460 -> [w469]
                      n213 = Build Array(w471) -> (w470:string[])
                      n214 = Bundle By Name(cluster=w469, "Tag"=w467) -> (w468:cluster{"Tag":string, "Parent tag":string})
                      n215 = call "change_ConfigDialog.vi"("tag and parent tag"=w468, "value"=w470, "Enum"=w472, "configtable"=w473) -> ("all device out"=w474:T2)  [unwired: 1 in, 6 out]
                    }
                  }
                }
              }
            }
          }
          event "LED": Value Change {
            n216 = event-data() -> ("CtlRef"=w480:refnum<vi>, "NewVal"=w478:bool)  [unwired: 5 out]
            n217 = call "chconfigset.vi"("Enum"=enum16{"init", "read", "treeheader", "ctrrefin"}."read") -> ("All ref"=w481:refnum<vi>[], "ref out"=w483:refnum<vi>[])  [unwired: 7 in, 2 out]
            n218 = property class="Tree (strict)"(reference=w489) -> (reference out=w488:refnum<vi>, "ActiveColNum"=w487:i32)  [unwired: 1 in, 1 out]
            n219 = Select(t="是", s=w478, f="否") -> (s? t:f=w475:string)
            n220 = Search 1D Array(1D array=w483, element=w480) -> (index of element=w486:i32)  [unwired: 1 in]
            n221 = Search 1D Array(1D array=w481, element=w480) -> (index of element=w479:i32)  [unwired: 1 in]
            n222 = Increment(x=w486) -> (x+1=w484:i32)
            n223 = Equal?(x=w487, y=w484) -> (x = y?=w485:bool)
            n224 = case shown="True" w485 {
              tunnel: w491 -> [w492 w495]
              tunnel: w475 -> [_ w503]
              tunnel: [w492 w494] -> w490
              tunnel: w488 -> [_ w502]
              tunnel: w479 -> [_ w493]
              frame False {
              }
              frame True {
                n225 = property class="Tree (strict)"(reference=w502, "Cell String"=w503) -> (reference out=w500:refnum<vi>, error out=w501:errorcluster)  [unwired: 1 in]
                n226 = call "get child tag.vi"("ChannalConfig"=w500, "error in (no error)"=w501) -> ("ChannalConfig out"=w497:refnum<vi>, "? parent"=w499:bool, "tag and parent tag"=w496:cluster{"Tag":string, "Parent tag":string}, "child tag"=w498:string[])  [unwired: 10 out]
                n227 = case shown="True" w499 {
                  tunnel: w497 -> [_ w516]
                  tunnel: w498 -> [_ w515]
                  tunnel: w503 -> [w509 w511]
                  tunnel: w496 -> [w507 w510]
                  tunnel: w495 -> [w506 w513]
                  tunnel: [w505 w514] -> w494
                  tunnel: w493 -> [w504 w512]
                  frame False {
                    n228 = Build Array(w509) -> (w508:string[])
                    n229 = call "change_ConfigDialog.vi"("tag and parent tag"=w507, "value"=w508, "Enum"=w504, "configtable"=w506) -> ("all device out"=w505:T2)  [unwired: 1 in, 6 out]
                  }
                  frame True {
                    n230 = call "chnage allchild cell.vi"("Active Cell:String"=w511, "all childtag"=w515, "ChannalConfig"=w516) -> ()  [unwired: 9 out]
                    n231 = for {
                      tunnel: w515 -> [w517] mode=indexing
                      shift-right: [w524] -> w514
                      shift-left: w513 -> [w523]
                      tunnel: w512 -> [w522]
                      tunnel: w511 -> [w521]
                      tunnel: w510 -> [w519]
                      n232 = Build Array(w521) -> (w520:string[])
                      n233 = Bundle By Name(cluster=w519, "Tag"=w517) -> (w518:cluster{"Tag":string, "Parent tag":string})
                      n234 = call "change_ConfigDialog.vi"("tag and parent tag"=w518, "value"=w520, "Enum"=w522, "configtable"=w523) -> ("all device out"=w524:T2)  [unwired: 1 in, 6 out]
                    }
                  }
                }
              }
            }
          }
          event Value Change {
            n235 = event-data() -> ("CtlRef"=w528:refnum<vi>, "NewVal"=w526:T1)  [unwired: 5 out]
            n236 = call "chconfigset.vi"("Enum"=enum16{"init", "read", "treeheader", "ctrrefin"}."read") -> ("All ref"=w530:refnum<vi>[], "ref out"=w532:refnum<vi>[])  [unwired: 7 in, 2 out]
            n237 = property class="Enum (strict)"(reference=w528) -> ("Strings []"=w527:string[])  [unwired: 1 in, 2 out]
            n238 = property class="Tree (strict)"(reference=w538) -> (reference out=w537:refnum<vi>, "ActiveColNum"=w536:i32)  [unwired: 1 in, 1 out]
            n239 = Search 1D Array(1D array=w530, element=w528) -> (index of element=w529:i32)  [unwired: 1 in]
            n240 = Search 1D Array(1D array=w532, element=w528) -> (index of element=w535:i32)  [unwired: 1 in]
            n241 = Index Array(array=w527, index=w526) -> (element=w525:string)
            n242 = Increment(x=w535) -> (x+1=w533:i32)
            n243 = Equal?(x=w536, y=w533) -> (x = y?=w534:bool)
            n244 = case shown="True" w534 {
              tunnel: w540 -> [w541 w544]
              tunnel: w525 -> [_ w552]
              tunnel: [w541 w543] -> w539
              tunnel: w537 -> [_ w551]
              tunnel: w529 -> [_ w542]
              frame False {
              }
              frame True {
                n245 = property class="Tree (strict)"(reference=w551, "Cell String"=w552) -> (reference out=w549:refnum<vi>, error out=w550:errorcluster)  [unwired: 1 in]
                n246 = call "get child tag.vi"("ChannalConfig"=w549, "error in (no error)"=w550) -> ("ChannalConfig out"=w546:refnum<vi>, "? parent"=w548:bool, "tag and parent tag"=w545:cluster{"Tag":string, "Parent tag":string}, "child tag"=w547:string[])  [unwired: 10 out]
                n247 = case shown="True" w548 {
                  tunnel: w546 -> [_ w565]
                  tunnel: w547 -> [_ w564]
                  tunnel: w552 -> [w558 w560]
                  tunnel: w545 -> [w556 w559]
                  tunnel: w544 -> [w555 w562]
                  tunnel: [w554 w563] -> w543
                  tunnel: w542 -> [w553 w561]
                  frame False {
                    n248 = Build Array(w558) -> (w557:string[])
                    n249 = call "change_ConfigDialog.vi"("tag and parent tag"=w556, "value"=w557, "Enum"=w553, "configtable"=w555) -> ("all device out"=w554:T2)  [unwired: 1 in, 6 out]
                  }
                  frame True {
                    n250 = call "chnage allchild cell.vi"("Active Cell:String"=w560, "all childtag"=w564, "ChannalConfig"=w565) -> ()  [unwired: 9 out]
                    n251 = for {
                      tunnel: w564 -> [w566] mode=indexing
                      shift-right: [w573] -> w563
                      shift-left: w562 -> [w572]
                      tunnel: w561 -> [w571]
                      tunnel: w560 -> [w570]
                      tunnel: w559 -> [w568]
                      n252 = Build Array(w570) -> (w569:string[])
                      n253 = Bundle By Name(cluster=w568, "Tag"=w566) -> (w567:cluster{"Tag":string, "Parent tag":string})
                      n254 = call "change_ConfigDialog.vi"("tag and parent tag"=w567, "value"=w569, "Enum"=w571, "configtable"=w572) -> ("all device out"=w573:T2)  [unwired: 1 in, 6 out]
                    }
                  }
                }
              }
            }
          }
          event Value Change {
            n255 = event-data() -> ("CtlRef"=w579:refnum<vi>, "NewVal"=w577:T6)  [unwired: 5 out]
            n256 = call "chconfigset.vi"("Enum"=enum16{"init", "read", "treeheader", "ctrrefin"}."read") -> ("All ref"=w580:refnum<vi>[], "ref out"=w582:refnum<vi>[])  [unwired: 7 in, 2 out]
            n257 = Unbundle By Name(w577) -> ("en"=w576:bool, "value"=w575:i32)
            n258 = property class="Tree (strict)"(reference=w588) -> (reference out=w587:refnum<vi>, "ActiveColNum"=w586:i32)  [unwired: 1 in, 1 out]
            n259 = case shown="False" w576 {
              tunnel: w575 -> [_ w595]
              tunnel: ["不滤波" w592] -> w574
              frame False {
              }
              frame True {
                n260 = Number To Decimal String(number=w595) -> (decimal integer string=w594:string)  [unwired: 1 in]
                n261 = Concatenate Strings(w594, "") -> (w592:string)
              }
            }
            n262 = Search 1D Array(1D array=w582, element=w579) -> (index of element=w585:i32)  [unwired: 1 in]
            n263 = Search 1D Array(1D array=w580, element=w579) -> (index of element=w578:i32)  [unwired: 1 in]
            n264 = Increment(x=w585) -> (x+1=w583:i32)
            n265 = Equal?(x=w586, y=w583) -> (x = y?=w584:bool)
            n266 = case shown="True" w584 {
              tunnel: w590 -> [w596 w599]
              tunnel: w574 -> [_ w607]
              tunnel: [w596 w598] -> w589
              tunnel: w587 -> [_ w606]
              tunnel: w578 -> [_ w597]
              frame False {
              }
              frame True {
                n267 = property class="Tree (strict)"(reference=w606, "Cell String"=w607) -> (reference out=w604:refnum<vi>, error out=w605:errorcluster)  [unwired: 1 in]
                n268 = call "get child tag.vi"("ChannalConfig"=w604, "error in (no error)"=w605) -> ("ChannalConfig out"=w601:refnum<vi>, "? parent"=w603:bool, "tag and parent tag"=w600:cluster{"Tag":string, "Parent tag":string}, "child tag"=w602:string[])  [unwired: 10 out]
                n269 = case shown="True" w603 {
                  tunnel: w601 -> [_ w620]
                  tunnel: w602 -> [_ w619]
                  tunnel: w607 -> [w613 w615]
                  tunnel: w600 -> [w611 w614]
                  tunnel: w599 -> [w610 w617]
                  tunnel: [w609 w618] -> w598
                  tunnel: w597 -> [w608 w616]
                  frame False {
                    n270 = Build Array(w613) -> (w612:string[])
                    n271 = call "change_ConfigDialog.vi"("tag and parent tag"=w611, "value"=w612, "Enum"=w608, "configtable"=w610) -> ("all device out"=w609:T2)  [unwired: 1 in, 6 out]
                  }
                  frame True {
                    n272 = call "chnage allchild cell.vi"("Active Cell:String"=w615, "all childtag"=w619, "ChannalConfig"=w620) -> ()  [unwired: 9 out]
                    n273 = for {
                      tunnel: w619 -> [w621] mode=indexing
                      shift-right: [w628] -> w618
                      shift-left: w617 -> [w627]
                      tunnel: w616 -> [w626]
                      tunnel: w615 -> [w625]
                      tunnel: w614 -> [w623]
                      n274 = Build Array(w625) -> (w624:string[])
                      n275 = Bundle By Name(cluster=w623, "Tag"=w621) -> (w622:cluster{"Tag":string, "Parent tag":string})
                      n276 = call "change_ConfigDialog.vi"("tag and parent tag"=w622, "value"=w624, "Enum"=w626, "configtable"=w627) -> ("all device out"=w628:T2)  [unwired: 1 in, 6 out]
                    }
                  }
                }
              }
            }
          }
          event Value Change {
            n277 = event-data() -> ("CtlRef"=w635:refnum<vi>, "NewVal"=w633:T5)  [unwired: 5 out]
            n278 = Unbundle By Name(w633) -> ("power_en"=w632:bool, "value"=w631:dbl, "Mode"=w629:enum16{"电压", "电流"})
            n279 = call "chconfigset.vi"("Enum"=enum16{"init", "read", "treeheader", "ctrrefin"}."read") -> ("All ref"=w636:refnum<vi>[], "ref out"=w638:refnum<vi>[])  [unwired: 7 in, 2 out]
            n280 = property class="Tree (strict)"(reference=w644) -> (reference out=w643:refnum<vi>, "ActiveColNum"=w642:i32)  [unwired: 1 in, 1 out]
            n281 = case shown="True" w632 {
              tunnel: w631 -> [_ w650]
              tunnel: ["无" w649] -> w630
              tunnel: w629 -> [_ w648]
              frame False {
              }
              frame True {
                n282 = case shown="\"电流\"" w648 {
                  tunnel: w650 -> [w654 w658]
                  tunnel: [w651 w655] -> w649
                  frame "电压", Default {
                    n283 = Number To Decimal String(number=w654) -> (decimal integer string=w653:string)  [unwired: 1 in]
                    n284 = Concatenate Strings(w653, "V") -> (w651:string)
                  }
                  frame "电流" {
                    n285 = Number To Fractional String(number=w658) -> (F-format string=w656:string)  [unwired: 3 in]
                    n286 = Concatenate Strings(w656, "mA") -> (w655:string)
                  }
                }
              }
            }
            n287 = Search 1D Array(1D array=w638, element=w635) -> (index of element=w641:i32)  [unwired: 1 in]
            n288 = Search 1D Array(1D array=w636, element=w635) -> (index of element=w634:i32)  [unwired: 1 in]
            n289 = Increment(x=w641) -> (x+1=w639:i32)
            n290 = Equal?(x=w642, y=w639) -> (x = y?=w640:bool)
            n291 = case shown="True" w640 {
              tunnel: w646 -> [w659 w662]
              tunnel: w630 -> [_ w670]
              tunnel: [w659 w661] -> w645
              tunnel: w643 -> [_ w669]
              tunnel: w634 -> [_ w660]
              frame False {
              }
              frame True {
                n292 = property class="Tree (strict)"(reference=w669, "Cell String"=w670) -> (reference out=w667:refnum<vi>, error out=w668:errorcluster)  [unwired: 1 in]
                n293 = call "get child tag.vi"("ChannalConfig"=w667, "error in (no error)"=w668) -> ("ChannalConfig out"=w664:refnum<vi>, "? parent"=w666:bool, "tag and parent tag"=w663:cluster{"Tag":string, "Parent tag":string}, "child tag"=w665:string[])  [unwired: 10 out]
                n294 = case shown="True" w666 {
                  tunnel: w664 -> [_ w683]
                  tunnel: w665 -> [_ w682]
                  tunnel: w670 -> [w676 w678]
                  tunnel: w663 -> [w674 w677]
                  tunnel: w662 -> [w673 w680]
                  tunnel: [w672 w681] -> w661
                  tunnel: w660 -> [w671 w679]
                  frame False {
                    n295 = Build Array(w676) -> (w675:string[])
                    n296 = call "change_ConfigDialog.vi"("tag and parent tag"=w674, "value"=w675, "Enum"=w671, "configtable"=w673) -> ("all device out"=w672:T2)  [unwired: 1 in, 6 out]
                  }
                  frame True {
                    n297 = call "chnage allchild cell.vi"("Active Cell:String"=w678, "all childtag"=w682, "ChannalConfig"=w683) -> ()  [unwired: 9 out]
                    n298 = for {
                      tunnel: w682 -> [w684] mode=indexing
                      shift-right: [w691] -> w681
                      shift-left: w680 -> [w690]
                      tunnel: w679 -> [w689]
                      tunnel: w678 -> [w688]
                      tunnel: w677 -> [w686]
                      n299 = Build Array(w688) -> (w687:string[])
                      n300 = Bundle By Name(cluster=w686, "Tag"=w684) -> (w685:cluster{"Tag":string, "Parent tag":string})
                      n301 = call "change_ConfigDialog.vi"("tag and parent tag"=w685, "value"=w687, "Enum"=w689, "configtable"=w690) -> ("all device out"=w691:T2)  [unwired: 1 in, 6 out]
                    }
                  }
                }
              }
            }
          }
          event "rate": Value Change {
            n302 = event-data() -> ("CtlRef"=w697:refnum<vi>, "NewVal"=w693:dbl)  [unwired: 5 out]
            n303 = call "chconfigset.vi"("Enum"=enum16{"init", "read", "treeheader", "ctrrefin"}."read") -> ("All ref"=w698:refnum<vi>[], "ref out"=w700:refnum<vi>[])  [unwired: 7 in, 2 out]
            n304 = Less?(x=w693, y=1000.0) -> (x < y?=w694:bool)
            n305 = case shown="False" w694 {
              tunnel: w693 -> [w710 w728]
              tunnel: [w709 w725] -> w692
              frame False {
                n306 = Less?(x=w710, y=1000000.0) -> (x < y?=w711:bool)
                n307 = case shown="False" w711 {
                  tunnel: w710 -> [w718 w724]
                  tunnel: [w714 w719] -> w709
                  frame False {
                    n308 = Divide(x=w718, y=1000000.0) -> (x/y=w716:dbl)
                    n309 = Number To Fractional String(number=w716) -> (F-format string=w715:string)  [unwired: 3 in]
                    n310 = Concatenate Strings(w715, "Mhz" ("string")) -> (w714:string)
                  }
                  frame True {
                    n311 = Divide(x=w724, y=1000.0) -> (x/y=w722:dbl)
                    n312 = Number To Fractional String(number=w722) -> (F-format string=w721:string)  [unwired: 3 in]
                    n313 = Concatenate Strings(w721, "kHz" ("string")) -> (w719:string)
                  }
                }
              }
              frame True {
                n314 = Number To Fractional String(number=w728) -> (F-format string=w727:string)  [unwired: 3 in]
                n315 = Concatenate Strings(w727, "Hz") -> (w725:string)
              }
            }
            n316 = property class="Tree (strict)"(reference=w706) -> (reference out=w705:refnum<vi>, "ActiveColNum"=w704:i32)  [unwired: 1 in, 1 out]
            n317 = Search 1D Array(1D array=w700, element=w697) -> (index of element=w703:i32)  [unwired: 1 in]
            n318 = Search 1D Array(1D array=w698, element=w697) -> (index of element=w696:i32)  [unwired: 1 in]
            n319 = Increment(x=w703) -> (x+1=w701:i32)
            n320 = Equal?(x=w704, y=w701) -> (x = y?=w702:bool)
            n321 = case shown="True" w702 {
              tunnel: w708 -> [w729 w732]
              tunnel: w692 -> [_ w740]
              tunnel: [w729 w731] -> w707
              tunnel: w705 -> [_ w739]
              tunnel: w696 -> [_ w730]
              frame False {
              }
              frame True {
                n322 = property class="Tree (strict)"(reference=w739, "Cell String"=w740) -> (reference out=w737:refnum<vi>, error out=w738:errorcluster)  [unwired: 1 in]
                n323 = call "get child tag.vi"("ChannalConfig"=w737, "error in (no error)"=w738) -> ("ChannalConfig out"=w734:refnum<vi>, "? parent"=w736:bool, "tag and parent tag"=w733:cluster{"Tag":string, "Parent tag":string}, "child tag"=w735:string[])  [unwired: 10 out]
                n324 = case shown="True" w736 {
                  tunnel: w734 -> [_ w753]
                  tunnel: w735 -> [_ w752]
                  tunnel: w740 -> [w746 w748]
                  tunnel: w733 -> [w744 w747]
                  tunnel: w732 -> [w743 w750]
                  tunnel: [w742 w751] -> w731
                  tunnel: w730 -> [w741 w749]
                  frame False {
                    n325 = Build Array(w746) -> (w745:string[])
                    n326 = call "change_ConfigDialog.vi"("tag and parent tag"=w744, "value"=w745, "Enum"=w741, "configtable"=w743) -> ("all device out"=w742:T2)  [unwired: 1 in, 6 out]
                  }
                  frame True {
                    n327 = call "chnage allchild cell.vi"("Active Cell:String"=w748, "all childtag"=w752, "ChannalConfig"=w753) -> ()  [unwired: 9 out]
                    n328 = for {
                      tunnel: w752 -> [w754] mode=indexing
                      shift-right: [w761] -> w751
                      shift-left: w750 -> [w760]
                      tunnel: w749 -> [w759]
                      tunnel: w748 -> [w758]
                      tunnel: w747 -> [w756]
                      n329 = Build Array(w758) -> (w757:string[])
                      n330 = Bundle By Name(cluster=w756, "Tag"=w754) -> (w755:cluster{"Tag":string, "Parent tag":string})
                      n331 = call "change_ConfigDialog.vi"("tag and parent tag"=w755, "value"=w757, "Enum"=w759, "configtable"=w760) -> ("all device out"=w761:T2)  [unwired: 1 in, 6 out]
                    }
                  }
                }
              }
            }
          }
          event "k", "b": Value Change {
            n332 = event-data() -> ("CtlRef"=w766:refnum<vi>, "NewVal"=w764:dbl)  [unwired: 5 out]
            n333 = Number To Fractional String(number=w764) -> (F-format string=w763:string)  [unwired: 3 in]
            n334 = call "chconfigset.vi"("Enum"=enum16{"init", "read", "treeheader", "ctrrefin"}."read") -> ("All ref"=w762:refnum<vi>[], "ref out"=w768:refnum<vi>[])  [unwired: 7 in, 2 out]
            n335 = property class="Tree (strict)"(reference=w774) -> (reference out=w773:refnum<vi>, "ActiveColNum"=w772:i32)  [unwired: 1 in, 1 out]
            n336 = Search 1D Array(1D array=w768, element=w766) -> (index of element=w771:i32)  [unwired: 1 in]
            n337 = Search 1D Array(1D array=w762, element=w766) -> (index of element=w765:i32)  [unwired: 1 in]
            n338 = Increment(x=w771) -> (x+1=w769:i32)
            n339 = Equal?(x=w772, y=w769) -> (x = y?=w770:bool)
            n340 = case shown="True" w770 {
              tunnel: w776 -> [w777 w780]
              tunnel: w763 -> [_ w788]
              tunnel: [w777 w779] -> w775
              tunnel: w773 -> [_ w787]
              tunnel: w765 -> [_ w778]
              frame False {
              }
              frame True {
                n341 = property class="Tree (strict)"(reference=w787, "Cell String"=w788) -> (reference out=w785:refnum<vi>, error out=w786:errorcluster)  [unwired: 1 in]
                n342 = call "get child tag.vi"("ChannalConfig"=w785, "error in (no error)"=w786) -> ("ChannalConfig out"=w782:refnum<vi>, "? parent"=w784:bool, "tag and parent tag"=w781:cluster{"Tag":string, "Parent tag":string}, "child tag"=w783:string[])  [unwired: 10 out]
                n343 = case shown="False" w784 {
                  tunnel: w782 -> [_ w801]
                  tunnel: w783 -> [_ w800]
                  tunnel: w788 -> [w794 w796]
                  tunnel: w781 -> [w792 w795]
                  tunnel: w780 -> [w791 w798]
                  tunnel: [w790 w799] -> w779
                  tunnel: w778 -> [w789 w797]
                  frame False {
                    n344 = Build Array(w794) -> (w793:string[])
                    n345 = call "change_ConfigDialog.vi"("tag and parent tag"=w792, "value"=w793, "Enum"=w789, "configtable"=w791) -> ("all device out"=w790:T2)  [unwired: 1 in, 6 out]
                  }
                  frame True {
                    n346 = call "chnage allchild cell.vi"("Active Cell:String"=w796, "all childtag"=w800, "ChannalConfig"=w801) -> ()  [unwired: 9 out]
                    n347 = for {
                      tunnel: w800 -> [w802] mode=indexing
                      shift-right: [w809] -> w799
                      shift-left: w798 -> [w808]
                      tunnel: w797 -> [w807]
                      tunnel: w796 -> [w806]
                      tunnel: w795 -> [w804]
                      n348 = Build Array(w806) -> (w805:string[])
                      n349 = Bundle By Name(cluster=w804, "Tag"=w802) -> (w803:cluster{"Tag":string, "Parent tag":string})
                      n350 = call "change_ConfigDialog.vi"("tag and parent tag"=w803, "value"=w805, "Enum"=w807, "configtable"=w808) -> ("all device out"=w809:T2)  [unwired: 1 in, 6 out]
                    }
                  }
                }
              }
            }
          }
          event Value Change {
            n351 = event-data() -> ("NewVal"=w811:T7)  [unwired: 2 out]
            n352 = control-ref of="Gain"() -> (w813:refnum<vi>)
            n353 = call "chconfigset.vi"("Enum"=enum16{"init", "read", "treeheader", "ctrrefin"}."read") -> ("All ref"=w815:refnum<vi>[], "ref out"=w817:refnum<vi>[])  [unwired: 7 in, 2 out]
            n354 = property class="Enum (strict)"(reference=w813) -> ("Strings []"=w812:string[])  [unwired: 1 in, 2 out]
            n355 = property class="Tree (strict)"(reference=w823) -> (reference out=w822:refnum<vi>, "ActiveColNum"=w821:i32)  [unwired: 1 in, 1 out]
            n356 = Search 1D Array(1D array=w817, element=w813) -> (index of element=w820:i32)  [unwired: 1 in]
            n357 = Search 1D Array(1D array=w815, element=w813) -> (index of element=w814:i32)  [unwired: 1 in]
            n358 = Index Array(array=w812, index=w811) -> (element=w810:string)
            n359 = Increment(x=w820) -> (x+1=w818:i32)
            n360 = Equal?(x=w821, y=w818) -> (x = y?=w819:bool)
            n361 = case shown="True" w819 {
              tunnel: w825 -> [w826 w829]
              tunnel: w810 -> [_ w837]
              tunnel: [w826 w828] -> w824
              tunnel: w822 -> [_ w836]
              tunnel: w814 -> [_ w827]
              frame False {
              }
              frame True {
                n362 = property class="Tree (strict)"(reference=w836, "Cell String"=w837) -> (reference out=w834:refnum<vi>, error out=w835:errorcluster)  [unwired: 1 in]
                n363 = call "get child tag.vi"("ChannalConfig"=w834, "error in (no error)"=w835) -> ("ChannalConfig out"=w831:refnum<vi>, "? parent"=w833:bool, "tag and parent tag"=w830:cluster{"Tag":string, "Parent tag":string}, "child tag"=w832:string[])  [unwired: 10 out]
                n364 = case shown="True" w833 {
                  tunnel: w831 -> [_ w850]
                  tunnel: w832 -> [_ w849]
                  tunnel: w837 -> [w843 w845]
                  tunnel: w830 -> [w841 w844]
                  tunnel: w829 -> [w840 w847]
                  tunnel: [w839 w848] -> w828
                  tunnel: w827 -> [w838 w846]
                  frame False {
                    n365 = Build Array(w843) -> (w842:string[])
                    n366 = call "change_ConfigDialog.vi"("tag and parent tag"=w841, "value"=w842, "Enum"=w838, "configtable"=w840) -> ("all device out"=w839:T2)  [unwired: 1 in, 6 out]
                  }
                  frame True {
                    n367 = call "chnage allchild cell.vi"("Active Cell:String"=w845, "all childtag"=w849, "ChannalConfig"=w850) -> ()  [unwired: 9 out]
                    n368 = for {
                      tunnel: w849 -> [w851] mode=indexing
                      shift-right: [w858] -> w848
                      shift-left: w847 -> [w857]
                      tunnel: w846 -> [w856]
                      tunnel: w845 -> [w855]
                      tunnel: w844 -> [w853]
                      n369 = Build Array(w855) -> (w854:string[])
                      n370 = Bundle By Name(cluster=w853, "Tag"=w851) -> (w852:cluster{"Tag":string, "Parent tag":string})
                      n371 = call "change_ConfigDialog.vi"("tag and parent tag"=w852, "value"=w854, "Enum"=w856, "configtable"=w857) -> ("all device out"=w858:T2)  [unwired: 1 in, 6 out]
                    }
                  }
                }
              }
            }
          }
          event "threshold": Value Change {
            n372 = event-data() -> ("OldVal"=w860:dbl)  [unwired: 3 out]
            n373 = control-ref of="Gain"() -> (w862:refnum<vi>)
            n374 = call "chconfigset.vi"("Enum"=enum16{"init", "read", "treeheader", "ctrrefin"}."read") -> ("All ref"=w864:refnum<vi>[], "ref out"=w866:refnum<vi>[])  [unwired: 7 in, 2 out]
            n375 = property class="Enum (strict)"(reference=w862) -> ("Strings []"=w861:string[])  [unwired: 1 in, 2 out]
            n376 = property class="Tree (strict)"(reference=w872) -> (reference out=w871:refnum<vi>, "ActiveColNum"=w870:i32)  [unwired: 1 in, 1 out]
            n377 = Search 1D Array(1D array=w866, element=w862) -> (index of element=w869:i32)  [unwired: 1 in]
            n378 = Search 1D Array(1D array=w864, element=w862) -> (index of element=w863:i32)  [unwired: 1 in]
            n379 = Index Array(array=w861, index=w860) -> (element=w859:string)
            n380 = Increment(x=w869) -> (x+1=w867:i32)
            n381 = Equal?(x=w870, y=w867) -> (x = y?=w868:bool)
            n382 = case shown="True" w868 {
              tunnel: w874 -> [w875 w878]
              tunnel: w859 -> [_ w886]
              tunnel: [w875 w877] -> w873
              tunnel: w871 -> [_ w885]
              tunnel: w863 -> [_ w876]
              frame False {
              }
              frame True {
                n383 = property class="Tree (strict)"(reference=w885, "Cell String"=w886) -> (reference out=w883:refnum<vi>, error out=w884:errorcluster)  [unwired: 1 in]
                n384 = call "get child tag.vi"("ChannalConfig"=w883, "error in (no error)"=w884) -> ("ChannalConfig out"=w880:refnum<vi>, "? parent"=w882:bool, "tag and parent tag"=w879:cluster{"Tag":string, "Parent tag":string}, "child tag"=w881:string[])  [unwired: 10 out]
                n385 = case shown="True" w882 {
                  tunnel: w880 -> [_ w899]
                  tunnel: w881 -> [_ w898]
                  tunnel: w886 -> [w892 w894]
                  tunnel: w879 -> [w890 w893]
                  tunnel: w878 -> [w889 w896]
                  tunnel: [w888 w897] -> w877
                  tunnel: w876 -> [w887 w895]
                  frame False {
                    n386 = Build Array(w892) -> (w891:string[])
                    n387 = call "change_ConfigDialog.vi"("tag and parent tag"=w890, "value"=w891, "Enum"=w887, "configtable"=w889) -> ("all device out"=w888:T2)  [unwired: 1 in, 6 out]
                  }
                  frame True {
                    n388 = call "chnage allchild cell.vi"("Active Cell:String"=w894, "all childtag"=w898, "ChannalConfig"=w899) -> ()  [unwired: 9 out]
                    n389 = for {
                      tunnel: w898 -> [w900] mode=indexing
                      shift-right: [w907] -> w897
                      shift-left: w896 -> [w906]
                      tunnel: w895 -> [w905]
                      tunnel: w894 -> [w904]
                      tunnel: w893 -> [w902]
                      n390 = Build Array(w904) -> (w903:string[])
                      n391 = Bundle By Name(cluster=w902, "Tag"=w900) -> (w901:cluster{"Tag":string, "Parent tag":string})
                      n392 = call "change_ConfigDialog.vi"("tag and parent tag"=w901, "value"=w903, "Enum"=w905, "configtable"=w906) -> ("all device out"=w907:T2)  [unwired: 1 in, 6 out]
                    }
                  }
                }
              }
            }
          }
          event "Etype": Value Change {
            n393 = event-data() -> ("CtlRef"=w909:refnum<vi>, "NewVal"=w908:string)  [unwired: 2 out]
            n394 = call "chconfigset.vi"("Enum"=enum16{"init", "read", "treeheader", "ctrrefin"}."read") -> ("All ref"=w911:refnum<vi>[], "ref out"=w913:refnum<vi>[])  [unwired: 7 in, 2 out]
            n395 = property class="Tree (strict)"(reference=w919) -> (reference out=w918:refnum<vi>, "ActiveColNum"=w917:i32)  [unwired: 1 in, 1 out]
            n396 = Search 1D Array(1D array=w913, element=w909) -> (index of element=w916:i32)  [unwired: 1 in]
            n397 = Search 1D Array(1D array=w911, element=w909) -> (index of element=w910:i32)  [unwired: 1 in]
            n398 = Increment(x=w916) -> (x+1=w914:i32)
            n399 = Equal?(x=w917, y=w914) -> (x = y?=w915:bool)
            n400 = case shown="True" w915 {
              tunnel: w921 -> [w922 w925]
              tunnel: w908 -> [_ w933]
              tunnel: [w922 w924] -> w920
              tunnel: w918 -> [_ w932]
              tunnel: w910 -> [_ w923]
              frame False {
              }
              frame True {
                n401 = property class="Tree (strict)"(reference=w932, "Cell String"=w933) -> (reference out=w930:refnum<vi>, error out=w931:errorcluster)  [unwired: 1 in]
                n402 = call "get child tag.vi"("ChannalConfig"=w930, "error in (no error)"=w931) -> ("ChannalConfig out"=w927:refnum<vi>, "? parent"=w929:bool, "tag and parent tag"=w926:cluster{"Tag":string, "Parent tag":string}, "child tag"=w928:string[])  [unwired: 10 out]
                n403 = case shown="True" w929 {
                  tunnel: w927 -> [_ w946]
                  tunnel: w928 -> [_ w945]
                  tunnel: w933 -> [w939 w941]
                  tunnel: w926 -> [w937 w940]
                  tunnel: w925 -> [w936 w943]
                  tunnel: [w935 w944] -> w924
                  tunnel: w923 -> [w934 w942]
                  frame False {
                    n404 = Build Array(w939) -> (w938:string[])
                    n405 = call "change_ConfigDialog.vi"("tag and parent tag"=w937, "value"=w938, "Enum"=w934, "configtable"=w936) -> ("all device out"=w935:T2)  [unwired: 1 in, 6 out]
                  }
                  frame True {
                    n406 = call "chnage allchild cell.vi"("Active Cell:String"=w941, "all childtag"=w945, "ChannalConfig"=w946) -> ()  [unwired: 9 out]
                    n407 = for {
                      tunnel: w945 -> [w947] mode=indexing
                      shift-right: [w954] -> w944
                      shift-left: w943 -> [w953]
                      tunnel: w942 -> [w952]
                      tunnel: w941 -> [w951]
                      tunnel: w940 -> [w949]
                      n408 = Build Array(w951) -> (w950:string[])
                      n409 = Bundle By Name(cluster=w949, "Tag"=w947) -> (w948:cluster{"Tag":string, "Parent tag":string})
                      n410 = call "change_ConfigDialog.vi"("tag and parent tag"=w948, "value"=w950, "Enum"=w952, "configtable"=w953) -> ("all device out"=w954:T2)  [unwired: 1 in, 6 out]
                    }
                  }
                }
              }
            }
          }
          event "sensorName": Value Change {
            n411 = event-data() -> ("CtlRef"=w960:refnum<vi>, "NewVal"=w967:string)  [unwired: 4 out]
            n412 = property class="Tree (strict)"(reference=w965) -> (reference out=w964:refnum<vi>, "ActiveColNum"=w963:i32)  [unwired: 1 in, 1 out]
            n413 = call "chconfigset.vi"("Enum"=enum16{"init", "read", "treeheader", "ctrrefin"}."read") -> ("ref out"=w956:refnum<vi>[])  [unwired: 7 in, 3 out]
            n414 = Search 1D Array(1D array=w956, element=w960) -> (index of element=w962:i32)  [unwired: 1 in]
            n415 = Increment(x=w962) -> (x+1=w958:i32)
            n416 = Equal?(x=w967, y="browse..." ("NewVal")) -> (x = y?=w969:bool)
            n417 = Equal?(x=w963, y=w958) -> (x = y?=w961:bool)
            n418 = case shown="True" w961 {
              tunnel: w969 -> [_ w980]
              tunnel: w968 -> [w971 w979]
              tunnel: w967 -> [_ w978]
              tunnel: [w971 w977] -> w966
              tunnel: w964 -> [_ w976]
              tunnel: w958 -> [_ w975]
              tunnel: w960 -> [_ w974]
              tunnel: w959 -> [_ w973]
              tunnel: w957 -> [_ w972]
              frame False {
              }
              frame True {
                n419 = case shown="False" w980 {
                  tunnel: w976 -> [w986 w1025]
                  tunnel: w978 -> [w989 _]
                  tunnel: w979 -> [w990 w1020]
                  tunnel: w975 -> [w991 w1026]
                  tunnel: w978 -> [_ _]
                  tunnel: [w981 w1028] -> w977
                  tunnel: w974 -> [_ w1024]
                  tunnel: w973 -> [_ w1023]
                  tunnel: w972 -> [_ w1021]
                  frame False {
                    w982 = i32[] [4, 5, 6, 7, 8]
                    n420 = disable-structure shown="Disabled" {
                      disable-tunnel: w990 -> [w998 _]
                      disable-tunnel: w989 -> [w997 _]
                      disable-tunnel: [w996 _] -> w988
                      disable-tunnel: [w995 _] -> w983
                      frame Disabled {
                        n421 = call "get senserdata.vi"("senser name"=w997, "configtable"=w998) -> ("CAl"=w996:T12, "sensers data"=w995:string[])  [unwired: 8 out]
                      }
                      frame Enabled {
                      }
                    }
                    n422 = for {
                      tunnel: [w1010] -> w985
                      tunnel: w989 -> [_]
                      tunnel: w986 -> [w1009]
                      tunnel: [w1007] -> w984
                      tunnel: w982 -> [w1006] mode=indexing
                      tunnel: w983 -> [w1005] mode=indexing
                      n423 = property class="Tree (strict)"(reference=w1009, "ActiveColNum"=w1006) -> (reference out=w1008:refnum<vi>)  [unwired: 1 in, 1 out]
                      n424 = property class="Tree (strict)"(reference=w1008, "Cell String"=w1005) -> (reference out=w1010:refnum<vi>, error out=w1007:errorcluster)  [unwired: 1 in]
                    }
                    n425 = call "get child tag.vi"("ChannalConfig"=w985, "error in (no error)"=w984) -> ("ChannalConfig out"=w987:refnum<vi>, "? parent"=w994:bool, "tag and parent tag"=w992:cluster{"Tag":string, "Parent tag":string}, "child tag"=w993:string[])  [unwired: 10 out]
                    n426 = disable-structure shown="Disabled" {
                      disable-tunnel: w992 -> [w1004 _]
                      disable-tunnel: w991 -> [w1003 _]
                      disable-tunnel: w990 -> [w1002 _]
                      disable-tunnel: w988 -> [w1001 _]
                      disable-tunnel: w983 -> [w1000 _]
                      disable-tunnel: [w999 _] -> w981
                      frame Disabled {
                        n427 = call "change_ConfigDialog.vi"("CAl"=w1001, "tag and parent tag"=w1004, "value"=w1000, "Enum"=w1003, "configtable"=w1002) -> ("all device out"=w999:T2)  [unwired: 6 out]
                      }
                      frame Enabled {
                      }
                    }
                    n428 = case shown="True" w994 {
                      tunnel: w993 -> [_ w1014]
                      tunnel: w989 -> [_ _]
                      tunnel: w987 -> [_ w1013]
                      tunnel: w983 -> [_ w1012]
                      tunnel: w982 -> [_ w1011]
                      frame False {
                      }
                      frame True {
                        n429 = for {
                          tunnel: w1014 -> [w1019]
                          tunnel: w1013 -> [w1018]
                          tunnel: w1012 -> [w1016] mode=indexing
                          tunnel: w1011 -> [w1015] mode=indexing
                          n430 = property class="Tree (strict)"(reference=w1018, "ActiveColNum"=w1015) -> (reference out=w1017:refnum<vi>)  [unwired: 1 in, 1 out]
                          n431 = call "chnage allchild cell.vi"("Active Cell:String"=w1016, "all childtag"=w1019, "ChannalConfig"=w1017) -> ()  [unwired: 9 out]
                        }
                      }
                    }
                  }
                  frame True {
                    n432 = disable-structure shown="Disabled" {
                      disable-tunnel: [w1033 _] -> w1027
                      disable-tunnel: w1023 -> [w1032 _]
                      disable-tunnel: [w1031 _] -> w1022
                      disable-tunnel: w1021 -> [w1030 _]
                      disable-tunnel: w1020 -> [w1029 _]
                      frame Disabled {
                        n433 = call "ConfigTransducer.vi"("configtable"=w1029, "Path"=w1032, "root path"=w1030) -> ("OK?"=w1031:bool, "select tr"=w1033:T13)
                      }
                      frame Enabled {
                      }
                    }
                    n434 = case shown="True" w1022 {
                      tunnel: w1020 -> [w1034 w1065]
                      tunnel: [w1034 w1040] -> w1028
                      tunnel: w1027 -> [_ w1038]
                      tunnel: w1026 -> [_ w1060]
                      tunnel: w1025 -> [_ w1058]
                      tunnel: w1024 -> [_ w1050]
                      frame False {
                      }
                      frame True {
                        w1051 = i32[] [4, 5, 6, 7, 8, 11]
                        n435 = Unbundle By Name(w1038) -> ("manner"=w1064:enum16{"线性", "查表"}, "data"=w1063:dbl[][], "sensorID"=w1045:string, "signal type"=w1039:string, "unit"=w1061:string)
                        n436 = call "computer max min & gains.vi"("Sensor"=w1038) -> ("gains"=w1035:string, "b value"=w1036:string, "k value"=w1037:string)  [unwired: 8 out]
                        n437 = Bundle("manner"=w1064, "data"=w1063) -> (w1062:T12)  [unwired: 1 out]
                        n438 = Build Array(w1045, w1039, w1061, w1037, w1036, w1035) -> (w1052:string[])
                        n439 = for {
                          tunnel: w1058 -> [w1090]
                          tunnel: [w1089] -> w1057
                          tunnel: [w1088] -> w1056
                          tunnel: w1052 -> [w1086] mode=indexing
                          tunnel: w1051 -> [w1085] mode=indexing
                          n440 = property class="Tree (strict)"(reference=w1090, "ActiveColNum"=w1085) -> (reference out=w1087:refnum<vi>)  [unwired: 1 in, 1 out]
                          n441 = property class="Tree (strict)"(reference=w1087, "Cell String"=w1086) -> (reference out=w1088:refnum<vi>, error out=w1089:errorcluster)  [unwired: 1 in]
                        }
                        n442 = call "get child tag.vi"("ChannalConfig"=w1056, "error in (no error)"=w1057) -> ("ChannalConfig out"=w1053:refnum<vi>, "? parent"=w1055:bool, "tag and parent tag"=w1059:cluster{"Tag":string, "Parent tag":string}, "child tag"=w1054:string[])  [unwired: 10 out]
                        n443 = case shown="True" w1055 {
                          tunnel: w1053 -> [_ w1075]
                          tunnel: w1054 -> [_ w1074]
                          tunnel: w1052 -> [_ w1073]
                          tunnel: w1051 -> [_ w1072]
                          frame False {
                          }
                          frame True {
                            n444 = for {
                              tunnel: w1075 -> [w1077]
                              tunnel: w1074 -> [w1080]
                              tunnel: w1073 -> [w1079] mode=indexing
                              tunnel: w1072 -> [w1078] mode=indexing
                              n445 = property class="Tree (strict)"(reference=w1077, "ActiveColNum"=w1078) -> (reference out=w1076:refnum<vi>)  [unwired: 1 in, 1 out]
                              n446 = call "chnage allchild cell.vi"("Active Cell:String"=w1079, "all childtag"=w1080, "ChannalConfig"=w1076) -> ()  [unwired: 9 out]
                            }
                          }
                        }
                        n447 = disable-structure shown="Disabled" {
                          disable-tunnel: w1065 -> [w1071 _]
                          disable-tunnel: w1062 -> [w1070 _]
                          disable-tunnel: w1060 -> [w1069 _]
                          disable-tunnel: w1059 -> [w1068 _]
                          disable-tunnel: w1052 -> [w1067 _]
                          disable-tunnel: [w1066 _] -> w1040
                          frame Disabled {
                            n448 = call "change_ConfigDialog.vi"("CAl"=w1070, "tag and parent tag"=w1068, "value"=w1067, "Enum"=w1069, "configtable"=w1071) -> ("all device out"=w1066:T2)  [unwired: 6 out]
                          }
                          frame Enabled {
                          }
                        }
                        n449 = property class="CmbBox"(reference=w1050, "Value"=w1045) -> (reference out=w1049:refnum<vi>, "Strings[]"=w1046:string[])  [unwired: 1 in, 1 out]
                        n450 = Search 1D Array(1D array=w1046, element=w1045) -> (index of element=w1048:i32)  [unwired: 1 in]
                        n451 = Equal?(x=w1048, y=-1) -> (x = y?=w1043:bool)
                        n452 = Not Equal?(x=w1045, y="") -> (x != y?=w1042:bool)
                        n453 = And(x=w1043, y=w1042) -> (x .and. y?=w1041:bool)
                        n454 = case shown="True" w1041 {
                          tunnel: w1049 -> [_ w1084]
                          tunnel: w1046 -> [_ w1082]
                          tunnel: w1045 -> [_ w1081]
                          frame False {
                          }
                          frame True {
                            n455 = Build Array (concatenate)(w1082, w1081) -> (w1083:string[])
                            n456 = property class="CmbBox"(reference=w1084, "Strings[]"=w1083) -> ()  [unwired: 1 in, 2 out]
                          }
                        }
                      }
                    }
                  }
                }
              }
            }
          }
          event "sensorName", "rate", "alarm", "enable", "ChannalName", "k", "b", "Etype": Mouse Leave {
            n457 = event-data() -> ("CtlRef"=w1093:refnum<vi>)  [unwired: 4 out]
            n458 = property class="Ctl"(reference=w1093, "Position"=T8 {"Left"=-200, "Top"=-200}) -> ()  [unwired: 1 in, 2 out]
          }
        }
      }
      "error out" <- w48
    }
  }
